vi "delme3.vi"() -> ()   [LabVIEW 2020]
uses:
  Project/GitInterface/Git-Repo JSON Typedef.ctl
panel:
  in  "Organization":string="P887"
  in  "Server":string="github.inbcu.com"
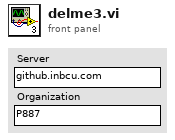
[diagram p1: front panel]
types:
  T1 = typedef "Git-Repo JSON Typedef.ctl" = cluster{"ID":string, "node_id":string, "name":string, "full_name":string, "private":string, "owner":string, "html_url":string, "description":string, "url":string, "collaborators_url":string, "teams_url":string}
  T2 = typedef "LabVIEWHTTPClient.lvlib/ClientHandle.ctl" = refnum<k1>
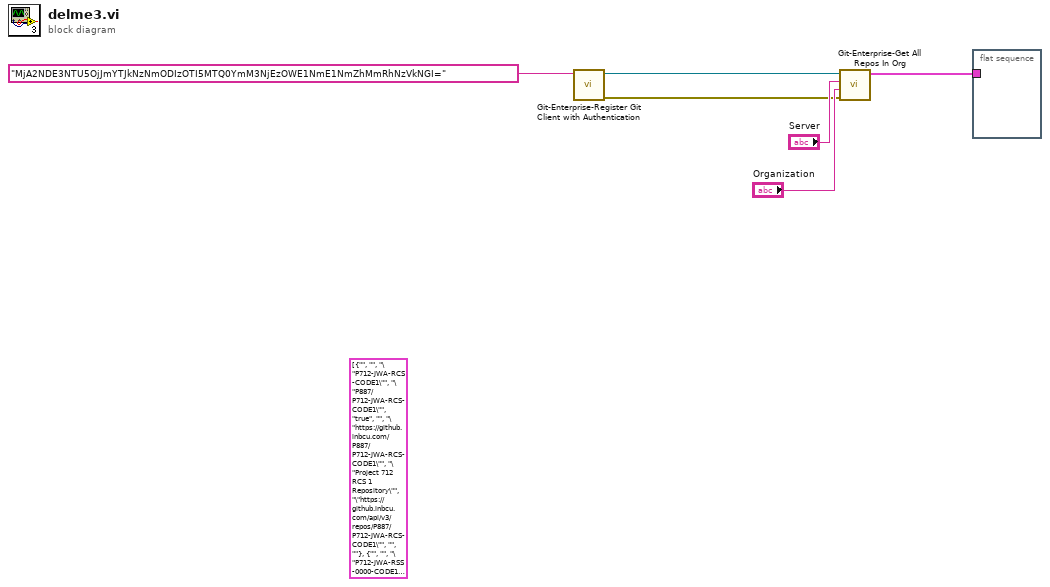
[diagram p0: block diagram]
diagram:
  (unwired) T1[] [{"ID"="", "node_id"="", "name"="\"P712-JWA-RCS-CODE1\"", "full_name"="\"P887/P712-JWA-RCS-CODE1\"", "private"="true", "owner"="", "html_url"="\"https://github.inbcu.com/P887/P712-JWA-RCS-CODE1\"", "description"="\"Project 712 RCS 1 Repository\"", "url"="\"https://github.inbcu.com/api/v3/repos/P887/P712-JWA-RCS-CODE1\"", "collaborators_url"="", "teams_url"=""}, {"ID"="", "node_id"="", "name"="\"P712-JWA-RSS-0000-CODE1\"", "full_name"="\"P887/P712-JWA-RSS-0000-CODE1\"", "private"="true", "owner"="", "html_url"="\"https://github.inbcu.com/P887/P712-JWA-RSS-0000-CODE1\"", "description"="\"RSS Software\"", "url"="\"https://github.inbcu.com/api/v3/repos/P887/P712-JWA-RSS-0000-CODE1\"", "collaborators_url"="", "teams_url"=""}, {"ID"="", "node_id"="", "name"="\"P714-KFP-RCS-CODE1\"", "full_name"="\"P887/P714-KFP-RCS-CODE1\"", "private"="true", "owner"="", "html_url"="\"https://github.inbcu.com/P887/P714-KFP-RCS-CODE1\"", "description"="\"KFP RCS Repository\"", "url"="\"https://github.inbcu.com/api/v3/repos/P887/P714-KFP-RCS-CODE1\"", "collaborators_url"="", "teams_url"=""}, {"ID"="", "node_id"="", "name"="\"P714-KFP-RSS-CODE1\"", "full_name"="\"P887/P714-KFP-RSS-CODE1\"", "private"="true", "owner"="", "html_url"="\"https://github.inbcu.com/P887/P714-KFP-RSS-CODE1\"", "description"="\"KFP RSS Software\"", "url"="\"https://github.inbcu.com/api/v3/repos/P887/P714-KFP-RSS-CODE1\"", "collaborators_url"="", "teams_url"=""}, {"ID"="", "node_id"="", "name"="\"P715-FJ-RCS-100-CODE1\"", "full_name"="\"P887/P715-FJ-RCS-100-CODE1\"", "private"="true", "owner"="", "html_url"="\"https://github.inbcu.com/P887/P715-FJ-RCS-100-CODE1\"", "description"="\"FJ RCS Software\"", "url"="\"https://github.inbcu.com/api/v3/repos/P887/P715-FJ-RCS-100-CODE1\"", "collaborators_url"="", "teams_url"=""}, {"ID"="", "node_id"="", "name"="\"P715-FJ-RSS-CODE1\"", "full_name"="\"P887/P715-FJ-RSS-CODE1\"", "private"="true", "owner"="", "html_url"="\"https://github.inbcu.com/P887/P715-FJ-RSS-CODE1\"", "description"="\"FJ RSS Software\"", "url"="\"https://github.inbcu.com/api/v3/repos/P887/P715-FJ-RSS-CODE1\"", "collaborators_url"="", "teams_url"=""}, {"ID"="", "node_id"="", "name"="\"P714-RIDE-AF-CODE1\"", "full_name"="\"P887/P714-RIDE-AF-CODE1\"", "private"="true", "owner"="", "html_url"="\"https://github.inbcu.com/P887/P714-RIDE-AF-CODE1\"", "description"="\"KFP Boat Ride SSC\"", "url"="\"https://github.inbcu.com/api/v3/repos/P887/P714-RIDE-AF-CODE1\"", "collaborators_url"="", "teams_url"=""}, {"ID"="", "node_id"="", "name"="\"P714-LAND-RSS-CODE1\"", "full_name"="\"P887/P714-LAND-RSS-CODE1\"", "private"="true", "owner"="", "html_url"="\"https://github.inbcu.com/P887/P714-LAND-RSS-CODE1\"", "description"="\"KFP Land RSS\"", "url"="\"https://github.inbcu.com/api/v3/repos/P887/P714-LAND-RSS-CODE1\"", "collaborators_url"="", "teams_url"=""}, {"ID"="", "node_id"="", "name"="\"P719-BARGE-SSC-CODE1\"", "full_name"="\"P887/P719-BARGE-SSC-CODE1\"", "private"="true", "owner"="", "html_url"="\"https://github.inbcu.com/P887/P719-BARGE-SSC-CODE1\"", "description"="\"Barge Controllers SSC\"", "url"="\"https://github.inbcu.com/api/v3/repos/P887/P719-BARGE-SSC-CODE1\"", "collaborators_url"="", "teams_url"=""}, {"ID"="", "node_id"="", "name"="\"LCA-RSS-CODE1\"", "full_name"="\"P887/LCA-RSS-CODE1\"", "private"="true", "owner"="", "html_url"="\"https://github.inbcu.com/P887/LCA-RSS-CODE1\"", "description"="\"LCA-RSS\"", "url"="\"https://github.inbcu.com/api/v3/repos/P887/LCA-RSS-CODE1\"", "collaborators_url"="", "teams_url"=""}, {"ID"="", "node_id"="", "name"="\"P717-COASTER-CODE1\"", "full_name"="\"P887/P717-COASTER-CODE1\"", "private"="true", "owner"="", "html_url"="\"https://github.inbcu.com/P887/P717-COASTER-CODE1\"", "description"="\"Pier Coaster RCS\"", "url"="\"https://github.inbcu.com/api/v3/repos/P887/P717-COASTER-CODE1\"", "collaborators_url"="", "teams_url"=""}, {"ID"="", "node_id"="", "name"="\"P717-PIER-ROUNDRIDE-CODE1\"", "full_name"="\"P887/P717-PIER-ROUNDRIDE-CODE1\"", "private"="true", "owner"="", "html_url"="\"https://github.inbcu.com/P887/P717-PIER-ROUNDRIDE-CODE1\"", "description"="\"P717 Pier Roundride\"", "url"="\"https://github.inbcu.com/api/v3/repos/P887/P717-PIER-ROUNDRIDE-CODE1\"", "collaborators_url"="", "teams_url"=""}, {"ID"="", "node_id"="", "name"="\"P717-MM-RCS-CODE1\"", "full_name"="\"P887/P717-MM-RCS-CODE1\"", "private"="true", "owner"="", "html_url"="\"https://github.inbcu.com/P887/P717-MM-RCS-CODE1\"", "description"="\"Minion Mayhem RCS Software\"", "url"="\"https://github.inbcu.com/api/v3/repos/P887/P717-MM-RCS-CODE1\"", "collaborators_url"="", "teams_url"=""}, {"ID"="", "node_id"="", "name"="\"P717-RSS-CODE1\"", "full_name"="\"P887/P717-RSS-CODE1\"", "private"="true", "owner"="", "html_url"="\"https://github.inbcu.com/P887/P717-RSS-CODE1\"", "description"="\"Minion Mayhem RSS Software\"", "url"="\"https://github.inbcu.com/api/v3/repos/P887/P717-RSS-CODE1\"", "collaborators_url"="", "teams_url"=""}, {"ID"="", "node_id"="", "name"="\"P717-HPU-CODE1\"", "full_name"="\"P887/P717-HPU-CODE1\"", "private"="true", "owner"="", "html_url"="\"https://github.inbcu.com/P887/P717-HPU-CODE1\"", "description"="\"Minion Mayhem HPU Software\"", "url"="\"https://github.inbcu.com/api/v3/repos/P887/P717-HPU-CODE1\"", "collaborators_url"="", "teams_url"=""}, {"ID"="", "node_id"="", "name"="\"P712-JFLYER-RCS-CODE1\"", "full_name"="\"P887/P712-JFLYER-RCS-CODE1\"", "private"="true", "owner"="", "html_url"="\"https://github.inbcu.com/P887/P712-JFLYER-RCS-CODE1\"", "description"="\"MACK Inverted Power Coaster\"", "url"="\"https://github.inbcu.com/api/v3/repos/P887/P712-JFLYER-RCS-CODE1\"", "collaborators_url"="", "teams_url"=""}, {"ID"="", "node_id"="", "name"="\"P716-TRANSFORMERS-RCS100-CODE1\"", "full_name"="\"P887/P716-TRANSFORMERS-RCS100-CODE1\"", "private"="true", "owner"="", "html_url"="\"https://github.inbcu.com/P887/P716-TRANSFORMERS-RCS100-CODE1\"", "description"="null", "url"="\"https://github.inbcu.com/api/v3/repos/P887/P716-TRANSFORMERS-RCS100-CODE1\"", "collaborators_url"="", "teams_url"=""}, {"ID"="", "node_id"="", "name"="\"P716-TRANSFORMERS-SSC400-CODE1\"", "full_name"="\"P887/P716-TRANSFORMERS-SSC400-CODE1\"", "private"="true", "owner"="", "html_url"="\"https://github.inbcu.com/P887/P716-TRANSFORMERS-SSC400-CODE1\"", "description"="null", "url"="\"https://github.inbcu.com/api/v3/repos/P887/P716-TRANSFORMERS-SSC400-CODE1\"", "collaborators_url"="", "teams_url"=""}, {"ID"="", "node_id"="", "name"="\"P716-TRANSFORMERS-SSC500-CODE1\"", "full_name"="\"P887/P716-TRANSFORMERS-SSC500-CODE1\"", "private"="true", "owner"="", "html_url"="\"https://github.inbcu.com/P887/P716-TRANSFORMERS-SSC500-CODE1\"", "description"="null", "url"="\"https://github.inbcu.com/api/v3/repos/P887/P716-TRANSFORMERS-SSC500-CODE1\"", "collaborators_url"="", "teams_url"=""}, {"ID"="", "node_id"="", "name"="\"P716-TRANSFORMERS-SSC600-CODE1\"", "full_name"="\"P887/P716-TRANSFORMERS-SSC600-CODE1\"", "private"="true", "owner"="", "html_url"="\"https://github.inbcu.com/P887/P716-TRANSFORMERS-SSC600-CODE1\"", "description"="null", "url"="\"https://github.inbcu.com/api/v3/repos/P887/P716-TRANSFORMERS-SSC600-CODE1\"", "collaborators_url"="", "teams_url"=""}, {"ID"="", "node_id"="", "name"="\"P716-TRANSFORMERS-SSC700-CODE1\"", "full_name"="\"P887/P716-TRANSFORMERS-SSC700-CODE1\"", "private"="true", "owner"="", "html_url"="\"https://github.inbcu.com/P887/P716-TRANSFORMERS-SSC700-CODE1\"", "description"="null", "url"="\"https://github.inbcu.com/api/v3/repos/P887/P716-TRANSFORMERS-SSC700-CODE1\"", "collaborators_url"="", "teams_url"=""}, {"ID"="", "node_id"="", "name"="\"P716-TRANSFORMERS-SSC800-CODE1\"", "full_name"="\"P887/P716-TRANSFORMERS-SSC800-CODE1\"", "private"="true", "owner"="", "html_url"="\"https://github.inbcu.com/P887/P716-TRANSFORMERS-SSC800-CODE1\"", "description"="null", "url"="\"https://github.inbcu.com/api/v3/repos/P887/P716-TRANSFORMERS-SSC800-CODE1\"", "collaborators_url"="", "teams_url"=""}, {"ID"="", "node_id"="", "name"="\"P716-TRANSFORMERS-SSC900-CODE1\"", "full_name"="\"P887/P716-TRANSFORMERS-SSC900-CODE1\"", "private"="true", "owner"="", "html_url"="\"https://github.inbcu.com/P887/P716-TRANSFORMERS-SSC900-CODE1\"", "description"="null", "url"="\"https://github.inbcu.com/api/v3/repos/P887/P716-TRANSFORMERS-SSC900-CODE1\"", "collaborators_url"="", "teams_url"=""}, {"ID"="", "node_id"="", "name"="\"P716-TRANSFORMERS-SSC1000-CODE1\"", "full_name"="\"P887/P716-TRANSFORMERS-SSC1000-CODE1\"", "private"="true", "owner"="", "html_url"="\"https://github.inbcu.com/P887/P716-TRANSFORMERS-SSC1000-CODE1\"", "description"="null", "url"="\"https://github.inbcu.com/api/v3/repos/P887/P716-TRANSFORMERS-SSC1000-CODE1\"", "collaborators_url"="", "teams_url"=""}, {"ID"="", "node_id"="", "name"="\"P716-TRANSFORMERS-SSC200-CODE1\"", "full_name"="\"P887/P716-TRANSFORMERS-SSC200-CODE1\"", "private"="true", "owner"="", "html_url"="\"https://github.inbcu.com/P887/P716-TRANSFORMERS-SSC200-CODE1\"", "description"="null", "url"="\"https://github.inbcu.com/api/v3/repos/P887/P716-TRANSFORMERS-SSC200-CODE1\"", "collaborators_url"="", "teams_url"=""}, {"ID"="", "node_id"="", "name"="\"P716-TRANSFORMERS-SSC300-CODE1\"", "full_name"="\"P887/P716-TRANSFORMERS-SSC300-CODE1\"", "private"="true", "owner"="", "html_url"="\"https://github.inbcu.com/P887/P716-TRANSFORMERS-SSC300-CODE1\"", "description"="null", "url"="\"https://github.inbcu.com/api/v3/repos/P887/P716-TRANSFORMERS-SSC300-CODE1\"", "collaborators_url"="", "teams_url"=""}, {"ID"="", "node_id"="", "name"="\"P715-LAND-LSS-CODE1\"", "full_name"="\"P887/P715-LAND-LSS-CODE1\"", "private"="true", "owner"="", "html_url"="\"https://github.inbcu.com/P887/P715-LAND-LSS-CODE1\"", "description"="null", "url"="\"https://github.inbcu.com/api/v3/repos/P887/P715-LAND-LSS-CODE1\"", "collaborators_url"="", "teams_url"=""}, {"ID"="", "node_id"="", "name"="\"P715-HIPPO-CODE1\"", "full_name"="\"P887/P715-HIPPO-CODE1\"", "private"="true", "owner"="", "html_url"="\"https://github.inbcu.com/P887/P715-HIPPO-CODE1\"", "description"="null", "url"="\"https://github.inbcu.com/api/v3/repos/P887/P715-HIPPO-CODE1\"", "collaborators_url"="", "teams_url"=""}, {"ID"="", "node_id"="", "name"="\"P711-FF-RCS-CODE1\"", "full_name"="\"P887/P711-FF-RCS-CODE1\"", "private"="true", "owner"="", "html_url"="\"https://github.inbcu.com/P887/P711-FF-RCS-CODE1\"", "description"="null", "url"="\"https://github.inbcu.com/api/v3/repos/P887/P711-FF-RCS-CODE1\"", "collaborators_url"="", "teams_url"=""}, {"ID"="", "node_id"="", "name"="\"P711-FF-RSS-CODE1\"", "full_name"="\"P887/P711-FF-RSS-CODE1\"", "private"="true", "owner"="", "html_url"="\"https://github.inbcu.com/P887/P711-FF-RSS-CODE1\"", "description"="null", "url"="\"https://github.inbcu.com/api/v3/repos/P887/P711-FF-RSS-CODE1\"", "collaborators_url"="", "teams_url"=""}, {"ID"="", "node_id"="", "name"="\"P712-JWA-RCS-CODE1\"", "full_name"="\"P887/P712-JWA-RCS-CODE1\"", "private"="true", "owner"="", "html_url"="\"https://github.inbcu.com/P887/P712-JWA-RCS-CODE1\"", "description"="\"Project 712 RCS 1 Repository\"", "url"="\"https://github.inbcu.com/api/v3/repos/P887/P712-JWA-RCS-CODE1\"", "collaborators_url"="", "teams_url"=""}, {"ID"="", "node_id"="", "name"="\"P712-JWA-RSS-0000-CODE1\"", "full_name"="\"P887/P712-JWA-RSS-0000-CODE1\"", "private"="true", "owner"="", "html_url"="\"https://github.inbcu.com/P887/P712-JWA-RSS-0000-CODE1\"", "description"="\"RSS Software\"", "url"="\"https://github.inbcu.com/api/v3/repos/P887/P712-JWA-RSS-0000-CODE1\"", "collaborators_url"="", "teams_url"=""}, {"ID"="", "node_id"="", "name"="\"P714-KFP-RCS-CODE1\"", "full_name"="\"P887/P714-KFP-RCS-CODE1\"", "private"="true", "owner"="", "html_url"="\"https://github.inbcu.com/P887/P714-KFP-RCS-CODE1\"", "description"="\"KFP RCS Repository\"", "url"="\"https://github.inbcu.com/api/v3/repos/P887/P714-KFP-RCS-CODE1\"", "collaborators_url"="", "teams_url"=""}, {"ID"="", "node_id"="", "name"="\"P714-KFP-RSS-CODE1\"", "full_name"="\"P887/P714-KFP-RSS-CODE1\"", "private"="true", "owner"="", "html_url"="\"https://github.inbcu.com/P887/P714-KFP-RSS-CODE1\"", "description"="\"KFP RSS Software\"", "url"="\"https://github.inbcu.com/api/v3/repos/P887/P714-KFP-RSS-CODE1\"", "collaborators_url"="", "teams_url"=""}, {"ID"="", "node_id"="", "name"="\"P715-FJ-RCS-100-CODE1\"", "full_name"="\"P887/P715-FJ-RCS-100-CODE1\"", "private"="true", "owner"="", "html_url"="\"https://github.inbcu.com/P887/P715-FJ-RCS-100-CODE1\"", "description"="\"FJ RCS Software\"", "url"="\"https://github.inbcu.com/api/v3/repos/P887/P715-FJ-RCS-100-CODE1\"", "collaborators_url"="", "teams_url"=""}, {"ID"="", "node_id"="", "name"="\"P715-FJ-RSS-CODE1\"", "full_name"="\"P887/P715-FJ-RSS-CODE1\"", "private"="true", "owner"="", "html_url"="\"https://github.inbcu.com/P887/P715-FJ-RSS-CODE1\"", "description"="\"FJ RSS Software\"", "url"="\"https://github.inbcu.com/api/v3/repos/P887/P715-FJ-RSS-CODE1\"", "collaborators_url"="", "teams_url"=""}, {"ID"="", "node_id"="", "name"="\"P714-RIDE-AF-CODE1\"", "full_name"="\"P887/P714-RIDE-AF-CODE1\"", "private"="true", "owner"="", "html_url"="\"https://github.inbcu.com/P887/P714-RIDE-AF-CODE1\"", "description"="\"KFP Boat Ride SSC\"", "url"="\"https://github.inbcu.com/api/v3/repos/P887/P714-RIDE-AF-CODE1\"", "collaborators_url"="", "teams_url"=""}, {"ID"="", "node_id"="", "name"="\"P714-LAND-RSS-CODE1\"", "full_name"="\"P887/P714-LAND-RSS-CODE1\"", "private"="true", "owner"="", "html_url"="\"https://github.inbcu.com/P887/P714-LAND-RSS-CODE1\"", "description"="\"KFP Land RSS\"", "url"="\"https://github.inbcu.com/api/v3/repos/P887/P714-LAND-RSS-CODE1\"", "collaborators_url"="", "teams_url"=""}, {"ID"="", "node_id"="", "name"="\"P719-BARGE-SSC-CODE1\"", "full_name"="\"P887/P719-BARGE-SSC-CODE1\"", "private"="true", "owner"="", "html_url"="\"https://github.inbcu.com/P887/P719-BARGE-SSC-CODE1\"", "description"="\"Barge Controllers SSC\"", "url"="\"https://github.inbcu.com/api/v3/repos/P887/P719-BARGE-SSC-CODE1\"", "collaborators_url"="", "teams_url"=""}, {"ID"="", "node_id"="", "name"="\"LCA-RSS-CODE1\"", "full_name"="\"P887/LCA-RSS-CODE1\"", "private"="true", "owner"="", "html_url"="\"https://github.inbcu.com/P887/LCA-RSS-CODE1\"", "description"="\"LCA-RSS\"", "url"="\"https://github.inbcu.com/api/v3/repos/P887/LCA-RSS-CODE1\"", "collaborators_url"="", "teams_url"=""}, {"ID"="", "node_id"="", "name"="\"P717-COASTER-CODE1\"", "full_name"="\"P887/P717-COASTER-CODE1\"", "private"="true", "owner"="", "html_url"="\"https://github.inbcu.com/P887/P717-COASTER-CODE1\"", "description"="\"Pier Coaster RCS\"", "url"="\"https://github.inbcu.com/api/v3/repos/P887/P717-COASTER-CODE1\"", "collaborators_url"="", "teams_url"=""}, {"ID"="", "node_id"="", "name"="\"P717-PIER-ROUNDRIDE-CODE1\"", "full_name"="\"P887/P717-PIER-ROUNDRIDE-CODE1\"", "private"="true", "owner"="", "html_url"="\"https://github.inbcu.com/P887/P717-PIER-ROUNDRIDE-CODE1\"", "description"="\"P717 Pier Roundride\"", "url"="\"https://github.inbcu.com/api/v3/repos/P887/P717-PIER-ROUNDRIDE-CODE1\"", "collaborators_url"="", "teams_url"=""}, {"ID"="", "node_id"="", "name"="\"P717-MM-RCS-CODE1\"", "full_name"="\"P887/P717-MM-RCS-CODE1\"", "private"="true", "owner"="", "html_url"="\"https://github.inbcu.com/P887/P717-MM-RCS-CODE1\"", "description"="\"Minion Mayhem RCS Software\"", "url"="\"https://github.inbcu.com/api/v3/repos/P887/P717-MM-RCS-CODE1\"", "collaborators_url"="", "teams_url"=""}, {"ID"="", "node_id"="", "name"="\"P717-RSS-CODE1\"", "full_name"="\"P887/P717-RSS-CODE1\"", "private"="true", "owner"="", "html_url"="\"https://github.inbcu.com/P887/P717-RSS-CODE1\"", "description"="\"Minion Mayhem RSS Software\"", "url"="\"https://github.inbcu.com/api/v3/repos/P887/P717-RSS-CODE1\"", "collaborators_url"="", "teams_url"=""}, {"ID"="", "node_id"="", "name"="\"P717-HPU-CODE1\"", "full_name"="\"P887/P717-HPU-CODE1\"", "private"="true", "owner"="", "html_url"="\"https://github.inbcu.com/P887/P717-HPU-CODE1\"", "description"="\"Minion Mayhem HPU Software\"", "url"="\"https://github.inbcu.com/api/v3/repos/P887/P717-HPU-CODE1\"", "collaborators_url"="", "teams_url"=""}, {"ID"="", "node_id"="", "name"="\"P712-JFLYER-RCS-CODE1\"", "full_name"="\"P887/P712-JFLYER-RCS-CODE1\"", "private"="true", "owner"="", "html_url"="\"https://github.inbcu.com/P887/P712-JFLYER-RCS-CODE1\"", "description"="\"MACK Inverted Power Coaster\"", "url"="\"https://github.inbcu.com/api/v3/repos/P887/P712-JFLYER-RCS-CODE1\"", "collaborators_url"="", "teams_url"=""}, {"ID"="", "node_id"="", "name"="\"P716-TRANSFORMERS-RCS100-CODE1\"", "full_name"="\"P887/P716-TRANSFORMERS-RCS100-CODE1\"", "private"="true", "owner"="", "html_url"="\"https://github.inbcu.com/P887/P716-TRANSFORMERS-RCS100-CODE1\"", "description"="null", "url"="\"https://github.inbcu.com/api/v3/repos/P887/P716-TRANSFORMERS-RCS100-CODE1\"", "collaborators_url"="", "teams_url"=""}, {"ID"="", "node_id"="", "name"="\"P716-TRANSFORMERS-SSC400-CODE1\"", "full_name"="\"P887/P716-TRANSFORMERS-SSC400-CODE1\"", "private"="true", "owner"="", "html_url"="\"https://github.inbcu.com/P887/P716-TRANSFORMERS-SSC400-CODE1\"", "description"="null", "url"="\"https://github.inbcu.com/api/v3/repos/P887/P716-TRANSFORMERS-SSC400-CODE1\"", "collaborators_url"="", "teams_url"=""}, {"ID"="", "node_id"="", "name"="\"P716-TRANSFORMERS-SSC500-CODE1\"", "full_name"="\"P887/P716-TRANSFORMERS-SSC500-CODE1\"", "private"="true", "owner"="", "html_url"="\"https://github.inbcu.com/P887/P716-TRANSFORMERS-SSC500-CODE1\"", "description"="null", "url"="\"https://github.inbcu.com/api/v3/repos/P887/P716-TRANSFORMERS-SSC500-CODE1\"", "collaborators_url"="", "teams_url"=""}, {"ID"="", "node_id"="", "name"="\"P716-TRANSFORMERS-SSC600-CODE1\"", "full_name"="\"P887/P716-TRANSFORMERS-SSC600-CODE1\"", "private"="true", "owner"="", "html_url"="\"https://github.inbcu.com/P887/P716-TRANSFORMERS-SSC600-CODE1\"", "description"="null", "url"="\"https://github.inbcu.com/api/v3/repos/P887/P716-TRANSFORMERS-SSC600-CODE1\"", "collaborators_url"="", "teams_url"=""}, {"ID"="", "node_id"="", "name"="\"P716-TRANSFORMERS-SSC700-CODE1\"", "full_name"="\"P887/P716-TRANSFORMERS-SSC700-CODE1\"", "private"="true", "owner"="", "html_url"="\"https://github.inbcu.com/P887/P716-TRANSFORMERS-SSC700-CODE1\"", "description"="null", "url"="\"https://github.inbcu.com/api/v3/repos/P887/P716-TRANSFORMERS-SSC700-CODE1\"", "collaborators_url"="", "teams_url"=""}, {"ID"="", "node_id"="", "name"="\"P716-TRANSFORMERS-SSC800-CODE1\"", "full_name"="\"P887/P716-TRANSFORMERS-SSC800-CODE1\"", "private"="true", "owner"="", "html_url"="\"https://github.inbcu.com/P887/P716-TRANSFORMERS-SSC800-CODE1\"", "description"="null", "url"="\"https://github.inbcu.com/api/v3/repos/P887/P716-TRANSFORMERS-SSC800-CODE1\"", "collaborators_url"="", "teams_url"=""}, {"ID"="", "node_id"="", "name"="\"P716-TRANSFORMERS-SSC900-CODE1\"", "full_name"="\"P887/P716-TRANSFORMERS-SSC900-CODE1\"", "private"="true", "owner"="", "html_url"="\"https://github.inbcu.com/P887/P716-TRANSFORMERS-SSC900-CODE1\"", "description"="null", "url"="\"https://github.inbcu.com/api/v3/repos/P887/P716-TRANSFORMERS-SSC900-CODE1\"", "collaborators_url"="", "teams_url"=""}, {"ID"="", "node_id"="", "name"="\"P716-TRANSFORMERS-SSC1000-CODE1\"", "full_name"="\"P887/P716-TRANSFORMERS-SSC1000-CODE1\"", "private"="true", "owner"="", "html_url"="\"https://github.inbcu.com/P887/P716-TRANSFORMERS-SSC1000-CODE1\"", "description"="null", "url"="\"https://github.inbcu.com/api/v3/repos/P887/P716-TRANSFORMERS-SSC1000-CODE1\"", "collaborators_url"="", "teams_url"=""}, {"ID"="", "node_id"="", "name"="\"P716-TRANSFORMERS-SSC200-CODE1\"", "full_name"="\"P887/P716-TRANSFORMERS-SSC200-CODE1\"", "private"="true", "owner"="", "html_url"="\"https://github.inbcu.com/P887/P716-TRANSFORMERS-SSC200-CODE1\"", "description"="null", "url"="\"https://github.inbcu.com/api/v3/repos/P887/P716-TRANSFORMERS-SSC200-CODE1\"", "collaborators_url"="", "teams_url"=""}, {"ID"="", "node_id"="", "name"="\"P716-TRANSFORMERS-SSC300-CODE1\"", "full_name"="\"P887/P716-TRANSFORMERS-SSC300-CODE1\"", "private"="true", "owner"="", "html_url"="\"https://github.inbcu.com/P887/P716-TRANSFORMERS-SSC300-CODE1\"", "description"="null", "url"="\"https://github.inbcu.com/api/v3/repos/P887/P716-TRANSFORMERS-SSC300-CODE1\"", "collaborators_url"="", "teams_url"=""}, {"ID"="", "node_id"="", "name"="\"P715-LAND-LSS-CODE1\"", "full_name"="\"P887/P715-LAND-LSS-CODE1\"", "private"="true", "owner"="", "html_url"="\"https://github.inbcu.com/P887/P715-LAND-LSS-CODE1\"", "description"="null", "url"="\"https://github.inbcu.com/api/v3/repos/P887/P715-LAND-LSS-CODE1\"", "collaborators_url"="", "teams_url"=""}, {"ID"="", "node_id"="", "name"="\"P715-HIPPO-CODE1\"", "full_name"="\"P887/P715-HIPPO-CODE1\"", "private"="true", "owner"="", "html_url"="\"https://github.inbcu.com/P887/P715-HIPPO-CODE1\"", "description"="null", "url"="\"https://github.inbcu.com/api/v3/repos/P887/P715-HIPPO-CODE1\"", "collaborators_url"="", "teams_url"=""}, {"ID"="", "node_id"="", "name"="\"P711-FF-RCS-CODE1\"", "full_name"="\"P887/P711-FF-RCS-CODE1\"", "private"="true", "owner"="", "html_url"="\"https://github.inbcu.com/P887/P711-FF-RCS-CODE1\"", "description"="null", "url"="\"https://github.inbcu.com/api/v3/repos/P887/P711-FF-RCS-CODE1\"", "collaborators_url"="", "teams_url"=""}, {"ID"="", "node_id"="", "name"="\"P711-FF-RSS-CODE1\"", "full_name"="\"P887/P711-FF-RSS-CODE1\"", "private"="true", "owner"="", "html_url"="\"https://github.inbcu.com/P887/P711-FF-RSS-CODE1\"", "description"="null", "url"="\"https://github.inbcu.com/api/v3/repos/P887/P711-FF-RSS-CODE1\"", "collaborators_url"="", "teams_url"=""}, {"ID"="", "node_id"="", "name"="\"P711-FF-HPU-CODE1\"", "full_name"="\"P887/P711-FF-HPU-CODE1\"", "private"="true", "owner"="", "html_url"="\"https://github.inbcu.com/P887/P711-FF-HPU-CODE1\"", "description"="null", "url"="\"https://github.inbcu.com/api/v3/repos/P887/P711-FF-HPU-CODE1\"", "collaborators_url"="", "teams_url"=""}, {"ID"="", "node_id"="", "name"="\"P711-FF-RVMV-CODE1\"", "full_name"="\"P887/P711-FF-RVMV-CODE1\"", "private"="true", "owner"="", "html_url"="\"https://github.inbcu.com/P887/P711-FF-RVMV-CODE1\"", "description"="null", "url"="\"https://github.inbcu.com/api/v3/repos/P887/P711-FF-RVMV-CODE1\"", "collaborators_url"="", "teams_url"=""}, {"ID"="", "node_id"="", "name"="\"P711-FF-SD-CODE1\"", "full_name"="\"P887/P711-FF-SD-CODE1\"", "private"="true", "owner"="", "html_url"="\"https://github.inbcu.com/P887/P711-FF-SD-CODE1\"", "description"="null", "url"="\"https://github.inbcu.com/api/v3/repos/P887/P711-FF-SD-CODE1\"", "collaborators_url"="", "teams_url"=""}, {"ID"="", "node_id"="", "name"="\"P711-FF-FS-CODE1\"", "full_name"="\"P887/P711-FF-FS-CODE1\"", "private"="true", "owner"="", "html_url"="\"https://github.inbcu.com/P887/P711-FF-FS-CODE1\"", "description"="\"Flying Screen\"", "url"="\"https://github.inbcu.com/api/v3/repos/P887/P711-FF-FS-CODE1\"", "collaborators_url"="", "teams_url"=""}, {"ID"="", "node_id"="", "name"="\"P711-FF-LN2-CODE1\"", "full_name"="\"P887/P711-FF-LN2-CODE1\"", "private"="true", "owner"="", "html_url"="\"https://github.inbcu.com/P887/P711-FF-LN2-CODE1\"", "description"="\"LN2\"", "url"="\"https://github.inbcu.com/api/v3/repos/P887/P711-FF-LN2-CODE1\"", "collaborators_url"="", "teams_url"=""}, {"ID"="", "node_id"="", "name"="\"P711-LCA-RSS100-CODE1\"", "full_name"="\"P887/P711-LCA-RSS100-CODE1\"", "private"="true", "owner"="", "html_url"="\"https://github.inbcu.com/P887/P711-LCA-RSS100-CODE1\"", "description"="null", "url"="\"https://github.inbcu.com/api/v3/repos/P887/P711-LCA-RSS100-CODE1\"", "collaborators_url"="", "teams_url"=""}, {"ID"="", "node_id"="", "name"="\"P711-MPT-RSS-CODE1\"", "full_name"="\"P887/P711-MPT-RSS-CODE1\"", "private"="true", "owner"="", "html_url"="\"https://github.inbcu.com/P887/P711-MPT-RSS-CODE1\"", "description"="null", "url"="\"https://github.inbcu.com/api/v3/repos/P887/P711-MPT-RSS-CODE1\"", "collaborators_url"="", "teams_url"=""}, {"ID"="", "node_id"="", "name"="\"P719-LAGOON-RSS-CODE1\"", "full_name"="\"P887/P719-LAGOON-RSS-CODE1\"", "private"="true", "owner"="", "html_url"="\"https://github.inbcu.com/P887/P719-LAGOON-RSS-CODE1\"", "description"="\"Lagoon Show RSS\"", "url"="\"https://github.inbcu.com/api/v3/repos/P887/P719-LAGOON-RSS-CODE1\"", "collaborators_url"="", "teams_url"=""}, {"ID"="", "node_id"="", "name"="\"P716-ROUNDRIDE-CODE1\"", "full_name"="\"P887/P716-ROUNDRIDE-CODE1\"", "private"="true", "owner"="", "html_url"="\"https://github.inbcu.com/P887/P716-ROUNDRIDE-CODE1\"", "description"="\"Transformers base Bumblebee Boogie Round Ride\"", "url"="\"https://github.inbcu.com/api/v3/repos/P887/P716-ROUNDRIDE-CODE1\"", "collaborators_url"="", "teams_url"=""}, {"ID"="", "node_id"="", "name"="\"P716-BBAF-CODE1\"", "full_name"="\"P887/P716-BBAF-CODE1\"", "private"="true", "owner"="", "html_url"="\"https://github.inbcu.com/P887/P716-BBAF-CODE1\"", "description"="\"Transformers Base Bumblebee Boogie Animated Figure\"", "url"="\"https://github.inbcu.com/api/v3/repos/P887/P716-BBAF-CODE1\"", "collaborators_url"="", "teams_url"=""}, {"ID"="", "node_id"="", "name"="\"P716-DECEPTICOASTER-RCS-CODE1\"", "full_name"="\"P887/P716-DECEPTICOASTER-RCS-CODE1\"", "private"="true", "owner"="", "html_url"="\"https://github.inbcu.com/P887/P716-DECEPTICOASTER-RCS-CODE1\"", "description"="\"Decepticoaster Ride System \"", "url"="\"https://github.inbcu.com/api/v3/repos/P887/P716-DECEPTICOASTER-RCS-CODE1\"", "collaborators_url"="", "teams_url"=""}, {"ID"="", "node_id"="", "name"="\"P714-12ARM-CODE1\"", "full_name"="\"P887/P714-12ARM-CODE1\"", "private"="true", "owner"="", "html_url"="\"https://github.inbcu.com/P887/P714-12ARM-CODE1\"", "description"="\"KFP Land 12 arm round ride\"", "url"="\"https://github.inbcu.com/api/v3/repos/P887/P714-12ARM-CODE1\"", "collaborators_url"="", "teams_url"=""}, {"ID"="", "node_id"="", "name"="\"P714-CAROUSEL-CODE1\"", "full_name"="\"P887/P714-CAROUSEL-CODE1\"", "private"="true", "owner"="", "html_url"="\"https://github.inbcu.com/P887/P714-CAROUSEL-CODE1\"", "description"="\"KFP Land Carousel Ride System\"", "url"="\"https://github.inbcu.com/api/v3/repos/P887/P714-CAROUSEL-CODE1\"", "collaborators_url"="", "teams_url"=""}, {"ID"="", "node_id"="", "name"="\"P716-DECEPTICOASTER-RSS-CODE1\"", "full_name"="\"P887/P716-DECEPTICOASTER-RSS-CODE1\"", "private"="true", "owner"="", "html_url"="\"https://github.inbcu.com/P887/P716-DECEPTICOASTER-RSS-CODE1\"", "description"="\"Transformers Decepticoaster RSS System\"", "url"="\"https://github.inbcu.com/api/v3/repos/P887/P716-DECEPTICOASTER-RSS-CODE1\"", "collaborators_url"="", "teams_url"=""}, {"ID"="", "node_id"="", "name"="\"P716-TRANSFORMERS-RSS-CODE1\"", "full_name"="\"P887/P716-TRANSFORMERS-RSS-CODE1\"", "private"="true", "owner"="", "html_url"="\"https://github.inbcu.com/P887/P716-TRANSFORMERS-RSS-CODE1\"", "description"="\"Transformers Ride RSS System\"", "url"="\"https://github.inbcu.com/api/v3/repos/P887/P716-TRANSFORMERS-RSS-CODE1\"", "collaborators_url"="", "teams_url"=""}, {"ID"="", "node_id"="", "name"="\"P715-FJ-RCS-200-CODE1\"", "full_name"="\"P887/P715-FJ-RCS-200-CODE1\"", "private"="true", "owner"="", "html_url"="\"https://github.inbcu.com/P887/P715-FJ-RCS-200-CODE1\"", "description"="null", "url"="\"https://github.inbcu.com/api/v3/repos/P887/P715-FJ-RCS-200-CODE1\"", "collaborators_url"="", "teams_url"=""}, {"ID"="", "node_id"="", "name"="\"P715-FJ-RCS-300-CODE1\"", "full_name"="\"P887/P715-FJ-RCS-300-CODE1\"", "private"="true", "owner"="", "html_url"="\"https://github.inbcu.com/P887/P715-FJ-RCS-300-CODE1\"", "description"="null", "url"="\"https://github.inbcu.com/api/v3/repos/P887/P715-FJ-RCS-300-CODE1\"", "collaborators_url"="", "teams_url"=""}, {"ID"="", "node_id"="", "name"="\"P715-FJ-RCS-400-CODE1\"", "full_name"="\"P887/P715-FJ-RCS-400-CODE1\"", "private"="true", "owner"="", "html_url"="\"https://github.inbcu.com/P887/P715-FJ-RCS-400-CODE1\"", "description"="\"TT (TT1 and TT2)\"", "url"="\"https://github.inbcu.com/api/v3/repos/P887/P715-FJ-RCS-400-CODE1\"", "collaborators_url"="", "teams_url"=""}, {"ID"="", "node_id"="", "name"="\"P715-FJ-RCS-500-CODE1\"", "full_name"="\"P887/P715-FJ-RCS-500-CODE1\"", "private"="true", "owner"="", "html_url"="\"https://github.inbcu.com/P887/P715-FJ-RCS-500-CODE1\"", "description"="\"PM (magic carpet)\"", "url"="\"https://github.inbcu.com/api/v3/repos/P887/P715-FJ-RCS-500-CODE1\"", "collaborators_url"="", "teams_url"=""}, {"ID"="", "node_id"="", "name"="\"P715-FJ-RCS-600-CODE1\"", "full_name"="\"P887/P715-FJ-RCS-600-CODE1\"", "private"="true", "owner"="", "html_url"="\"https://github.inbcu.com/P887/P715-FJ-RCS-600-CODE1\"", "description"="\"WSS\"", "url"="\"https://github.inbcu.com/api/v3/repos/P887/P715-FJ-RCS-600-CODE1\"", "collaborators_url"="", "teams_url"=""}, {"ID"="", "node_id"="", "name"="\"P715-FJ-VCS-1-CODE1\"", "full_name"="\"P887/P715-FJ-VCS-1-CODE1\"", "private"="true", "owner"="", "html_url"="\"https://github.inbcu.com/P887/P715-FJ-VCS-1-CODE1\"", "description"="\"VCS 1\"", "url"="\"https://github.inbcu.com/api/v3/repos/P887/P715-FJ-VCS-1-CODE1\"", "collaborators_url"="", "teams_url"=""}, {"ID"="", "node_id"="", "name"="\"P715-FJ-SSC-700-CODE1\"", "full_name"="\"P887/P715-FJ-SSC-700-CODE1\"", "private"="true", "owner"="", "html_url"="\"https://github.inbcu.com/P887/P715-FJ-SSC-700-CODE1\"", "description"="\"Carousel 1\"", "url"="\"https://github.inbcu.com/api/v3/repos/P887/P715-FJ-SSC-700-CODE1\"", "collaborators_url"="", "teams_url"=""}, {"ID"="", "node_id"="", "name"="\"P715-FJ-SSC-800-CODE1\"", "full_name"="\"P887/P715-FJ-SSC-800-CODE1\"", "private"="true", "owner"="", "html_url"="\"https://github.inbcu.com/P887/P715-FJ-SSC-800-CODE1\"", "description"="\"Carousel 2\"", "url"="\"https://github.inbcu.com/api/v3/repos/P887/P715-FJ-SSC-800-CODE1\"", "collaborators_url"="", "teams_url"=""}, {"ID"="", "node_id"="", "name"="\"P715-FJ-SSC-900-CODE1\"", "full_name"="\"P887/P715-FJ-SSC-900-CODE1\"", "private"="true", "owner"="", "html_url"="\"https://github.inbcu.com/P887/P715-FJ-SSC-900-CODE1\"", "description"="\"Carousel 3\"", "url"="\"https://github.inbcu.com/api/v3/repos/P887/P715-FJ-SSC-900-CODE1\"", "collaborators_url"="", "teams_url"=""}, {"ID"="", "node_id"="", "name"="\"P715-FJ-SSC-1000-CODE1\"", "full_name"="\"P887/P715-FJ-SSC-1000-CODE1\"", "private"="true", "owner"="", "html_url"="\"https://github.inbcu.com/P887/P715-FJ-SSC-1000-CODE1\"", "description"="\"Dementor Willow SAE\"", "url"="\"https://github.inbcu.com/api/v3/repos/P887/P715-FJ-SSC-1000-CODE1\"", "collaborators_url"="", "teams_url"=""}, {"ID"="", "node_id"="", "name"="\"P715-FJ-SSC-2100-CODE1\"", "full_name"="\"P887/P715-FJ-SSC-2100-CODE1\"", "private"="true", "owner"="", "html_url"="\"https://github.inbcu.com/P887/P715-FJ-SSC-2100-CODE1\"", "description"="\"Dragon\"", "url"="\"https://github.inbcu.com/api/v3/repos/P887/P715-FJ-SSC-2100-CODE1\"", "collaborators_url"="", "teams_url"=""}, {"ID"="", "node_id"="", "name"="\"P715-FJ-SSC-1200-CODE1\"", "full_name"="\"P887/P715-FJ-SSC-1200-CODE1\"", "private"="true", "owner"="", "html_url"="\"https://github.inbcu.com/P887/P715-FJ-SSC-1200-CODE1\"", "description"="\"Scene 1 - 7 Special Effects\"", "url"="\"https://github.inbcu.com/api/v3/repos/P887/P715-FJ-SSC-1200-CODE1\"", "collaborators_url"="", "teams_url"=""}, {"ID"="", "node_id"="", "name"="\"P715-FJ-SSC-1300-CODE1\"", "full_name"="\"P887/P715-FJ-SSC-1300-CODE1\"", "private"="true", "owner"="", "html_url"="\"https://github.inbcu.com/P887/P715-FJ-SSC-1300-CODE1\"", "description"="\"Scene 8-11 Special Effects\"", "url"="\"https://github.inbcu.com/api/v3/repos/P887/P715-FJ-SSC-1300-CODE1\"", "collaborators_url"="", "teams_url"=""}, {"ID"="", "node_id"="", "name"="\"P712-JWA-TS-CODE1\"", "full_name"="\"P887/P712-JWA-TS-CODE1\"", "private"="true", "owner"="", "html_url"="\"https://github.inbcu.com/P887/P712-JWA-TS-CODE1\"", "description"="\"JW TS RCS 200\"", "url"="\"https://github.inbcu.com/api/v3/repos/P887/P712-JWA-TS-CODE1\"", "collaborators_url"="", "teams_url"=""}, {"ID"="", "node_id"="", "name"="\"P712-JWA-SSC-2100-IREX1-CODE1\"", "full_name"="\"P887/P712-JWA-SSC-2100-IREX1-CODE1\"", "private"="true", "owner"="", "html_url"="\"https://github.inbcu.com/P887/P712-JWA-SSC-2100-IREX1-CODE1\"", "description"="\"JW Large AF SSC 2100\"", "url"="\"https://github.inbcu.com/api/v3/repos/P887/P712-JWA-SSC-2100-IREX1-CODE1\"", "collaborators_url"="", "teams_url"=""}, {"ID"="", "node_id"="", "name"="\"P712-JWA-SSC-2200-Anky-CODE1\"", "full_name"="\"P887/P712-JWA-SSC-2200-Anky-CODE1\"", "private"="true", "owner"="", "html_url"="\"https://github.inbcu.com/P887/P712-JWA-SSC-2200-Anky-CODE1\"", "description"="\"JW Large AF SSC 2200\"", "url"="\"https://github.inbcu.com/api/v3/repos/P887/P712-JWA-SSC-2200-Anky-CODE1\"", "collaborators_url"="", "teams_url"=""}, {"ID"="", "node_id"="", "name"="\"P712-JWA-SSC-2300-IREX2-CODE1\"", "full_name"="\"P887/P712-JWA-SSC-2300-IREX2-CODE1\"", "private"="true", "owner"="", "html_url"="\"https://github.inbcu.com/P887/P712-JWA-SSC-2300-IREX2-CODE1\"", "description"="\"JW Large AF SSC 2300\"", "url"="\"https://github.inbcu.com/api/v3/repos/P887/P712-JWA-SSC-2300-IREX2-CODE1\"", "collaborators_url"="", "teams_url"=""}, {"ID"="", "node_id"="", "name"="\"P712-JWA-SSC-2700-IREX3-CODE1\"", "full_name"="\"P887/P712-JWA-SSC-2700-IREX3-CODE1\"", "private"="true", "owner"="", "html_url"="\"https://github.inbcu.com/P887/P712-JWA-SSC-2700-IREX3-CODE1\"", "description"="\"JW Large AF SSC 2700\"", "url"="\"https://github.inbcu.com/api/v3/repos/P887/P712-JWA-SSC-2700-IREX3-CODE1\"", "collaborators_url"="", "teams_url"=""}, {"ID"="", "node_id"="", "name"="\"P712-JWA-SSC-2800-TREX-CODE1\"", "full_name"="\"P887/P712-JWA-SSC-2800-TREX-CODE1\"", "private"="true", "owner"="", "html_url"="\"https://github.inbcu.com/P887/P712-JWA-SSC-2800-TREX-CODE1\"", "description"="\"JW Large AF SSC 2800\"", "url"="\"https://github.inbcu.com/api/v3/repos/P887/P712-JWA-SSC-2800-TREX-CODE1\"", "collaborators_url"="", "teams_url"=""}, {"ID"="", "node_id"="", "name"="\"P712-JWA-SSC-2900-FH-CODE1\"", "full_name"="\"P887/P712-JWA-SSC-2900-FH-CODE1\"", "private"="true", "owner"="", "html_url"="\"https://github.inbcu.com/P887/P712-JWA-SSC-2900-FH-CODE1\"", "description"="\"JW Large AF SSC 2900\"", "url"="\"https://github.inbcu.com/api/v3/repos/P887/P712-JWA-SSC-2900-FH-CODE1\"", "collaborators_url"="", "teams_url"=""}, {"ID"="", "node_id"="", "name"="\"P712-JW-SSC-2400-CODE1\"", "full_name"="\"P887/P712-JW-SSC-2400-CODE1\"", "private"="true", "owner"="", "html_url"="\"https://github.inbcu.com/P887/P712-JW-SSC-2400-CODE1\"", "description"="\"JW SAE\"", "url"="\"https://github.inbcu.com/api/v3/repos/P887/P712-JW-SSC-2400-CODE1\"", "collaborators_url"="", "teams_url"=""}, {"ID"="", "node_id"="", "name"="\"P712-JW-SSC-2600-CODE1\"", "full_name"="\"P887/P712-JW-SSC-2600-CODE1\"", "private"="true", "owner"="", "html_url"="\"https://github.inbcu.com/P887/P712-JW-SSC-2600-CODE1\"", "description"="\"JW Raptor\"", "url"="\"https://github.inbcu.com/api/v3/repos/P887/P712-JW-SSC-2600-CODE1\"", "collaborators_url"="", "teams_url"=""}, {"ID"="", "node_id"="", "name"="\"P712-JW-SSC-2500-CODE1\"", "full_name"="\"P887/P712-JW-SSC-2500-CODE1\"", "private"="true", "owner"="", "html_url"="\"https://github.inbcu.com/P887/P712-JW-SSC-2500-CODE1\"", "description"="\"JW SA\"", "url"="\"https://github.inbcu.com/api/v3/repos/P887/P712-JW-SSC-2500-CODE1\"", "collaborators_url"="", "teams_url"=""}, {"ID"="", "node_id"="", "name"="\"P712-JWA-SCS-2000-CODE1\"", "full_name"="\"P887/P712-JWA-SCS-2000-CODE1\"", "private"="true", "owner"="", "html_url"="\"https://github.inbcu.com/P887/P712-JWA-SCS-2000-CODE1\"", "description"="\"JW SCS\"", "url"="\"https://github.inbcu.com/api/v3/repos/P887/P712-JWA-SCS-2000-CODE1\"", "collaborators_url"="", "teams_url"=""}, {"ID"="", "node_id"="", "name"="\"P712-JWA-VCS-CODE1\"", "full_name"="\"P887/P712-JWA-VCS-CODE1\"", "private"="true", "owner"="", "html_url"="\"https://github.inbcu.com/P887/P712-JWA-VCS-CODE1\"", "description"="\"JW VCS 1\"", "url"="\"https://github.inbcu.com/api/v3/repos/P887/P712-JWA-VCS-CODE1\"", "collaborators_url"="", "teams_url"=""}, {"ID"="", "node_id"="", "name"="\"P711-LCA-SSC200-CODE1\"", "full_name"="\"P887/P711-LCA-SSC200-CODE1\"", "private"="true", "owner"="", "html_url"="\"https://github.inbcu.com/P887/P711-LCA-SSC200-CODE1\"", "description"="\"Lights Camera Action SAE/SFX SSC\"", "url"="\"https://github.inbcu.com/api/v3/repos/P887/P711-LCA-SSC200-CODE1\"", "collaborators_url"="", "teams_url"=""}, {"ID"="", "node_id"="", "name"="\"P711-LCA-SSC300-CODE1\"", "full_name"="\"P887/P711-LCA-SSC300-CODE1\"", "private"="true", "owner"="", "html_url"="\"https://github.inbcu.com/P887/P711-LCA-SSC300-CODE1\"", "description"="\"Lights Camera Action SAE/SFX SSC\"", "url"="\"https://github.inbcu.com/api/v3/repos/P887/P711-LCA-SSC300-CODE1\"", "collaborators_url"="", "teams_url"=""}, {"ID"="", "node_id"="", "name"="\"P711-LCA-SSC400-CODE1\"", "full_name"="\"P887/P711-LCA-SSC400-CODE1\"", "private"="true", "owner"="", "html_url"="\"https://github.inbcu.com/P887/P711-LCA-SSC400-CODE1\"", "description"="\"Lights Camera Action SAE/SFX SSC\"", "url"="\"https://github.inbcu.com/api/v3/repos/P887/P711-LCA-SSC400-CODE1\"", "collaborators_url"="", "teams_url"=""}, {"ID"="", "node_id"="", "name"="\"P711-LCA-SSC500-CODE1\"", "full_name"="\"P887/P711-LCA-SSC500-CODE1\"", "private"="true", "owner"="", "html_url"="\"https://github.inbcu.com/P887/P711-LCA-SSC500-CODE1\"", "description"="\"Lights Camera Action SAE/SFX SSC\"", "url"="\"https://github.inbcu.com/api/v3/repos/P887/P711-LCA-SSC500-CODE1\"", "collaborators_url"="", "teams_url"=""}, {"ID"="", "node_id"="", "name"="\"P711-LCA-SSC600-CODE1\"", "full_name"="\"P887/P711-LCA-SSC600-CODE1\"", "private"="true", "owner"="", "html_url"="\"https://github.inbcu.com/P887/P711-LCA-SSC600-CODE1\"", "description"="\"Lights Camera Action SAE/SFX SSC\"", "url"="\"https://github.inbcu.com/api/v3/repos/P887/P711-LCA-SSC600-CODE1\"", "collaborators_url"="", "teams_url"=""}, {"ID"="", "node_id"="", "name"="\"P711-LCA-SSC700-CODE1\"", "full_name"="\"P887/P711-LCA-SSC700-CODE1\"", "private"="true", "owner"="", "html_url"="\"https://github.inbcu.com/P887/P711-LCA-SSC700-CODE1\"", "description"="\"Lights Camera Action SAE/SFX SSC\"", "url"="\"https://github.inbcu.com/api/v3/repos/P887/P711-LCA-SSC700-CODE1\"", "collaborators_url"="", "teams_url"=""}, {"ID"="", "node_id"="", "name"="\"P711-LCA-FSC800-CODE1\"", "full_name"="\"P887/P711-LCA-FSC800-CODE1\"", "private"="true", "owner"="", "html_url"="\"https://github.inbcu.com/P887/P711-LCA-FSC800-CODE1\"", "description"="null", "url"="\"https://github.inbcu.com/api/v3/repos/P887/P711-LCA-FSC800-CODE1\"", "collaborators_url"="", "teams_url"=""}, {"ID"="", "node_id"="", "name"="\"P715-LAND-AF-SSC1200-CODE1\"", "full_name"="\"P887/P715-LAND-AF-SSC1200-CODE1\"", "private"="true", "owner"="", "html_url"="\"https://github.inbcu.com/P887/P715-LAND-AF-SSC1200-CODE1\"", "description"="\"Cinnabar\"", "url"="\"https://github.inbcu.com/api/v3/repos/P887/P715-LAND-AF-SSC1200-CODE1\"", "collaborators_url"="", "teams_url"=""}, {"ID"="", "node_id"="", "name"="\"P715-LAND-AF-SSC1400-CODE1\"", "full_name"="\"P887/P715-LAND-AF-SSC1400-CODE1\"", "private"="true", "owner"="", "html_url"="\"https://github.inbcu.com/P887/P715-LAND-AF-SSC1400-CODE1\"", "description"="\"Cinnabar\"", "url"="\"https://github.inbcu.com/api/v3/repos/P887/P715-LAND-AF-SSC1400-CODE1\"", "collaborators_url"="", "teams_url"=""}, {"ID"="", "node_id"="", "name"="\"P715-501A-SSC-0200-CODE1\"", "full_name"="\"P887/P715-501A-SSC-0200-CODE1\"", "private"="true", "owner"="", "html_url"="\"https://github.inbcu.com/P887/P715-501A-SSC-0200-CODE1\"", "description"="\"Cinnabar\"", "url"="\"https://github.inbcu.com/api/v3/repos/P887/P715-501A-SSC-0200-CODE1\"", "collaborators_url"="", "teams_url"=""}, {"ID"="", "node_id"="", "name"="\"P715-501A-SSC-0300-CODE1\"", "full_name"="\"P887/P715-501A-SSC-0300-CODE1\"", "private"="true", "owner"="", "html_url"="\"https://github.inbcu.com/P887/P715-501A-SSC-0300-CODE1\"", "description"="\"Cinnabar\"", "url"="\"https://github.inbcu.com/api/v3/repos/P887/P715-501A-SSC-0300-CODE1\"", "collaborators_url"="", "teams_url"=""}, {"ID"="", "node_id"="", "name"="\"P715-506-SSC-0400-CODE1\"", "full_name"="\"P887/P715-506-SSC-0400-CODE1\"", "private"="true", "owner"="", "html_url"="\"https://github.inbcu.com/P887/P715-506-SSC-0400-CODE1\"", "description"="\"Cinnabar\"", "url"="\"https://github.inbcu.com/api/v3/repos/P887/P715-506-SSC-0400-CODE1\"", "collaborators_url"="", "teams_url"=""}, {"ID"="", "node_id"="", "name"="\"P715-501B-SSC-1200-CODE1\"", "full_name"="\"P887/P715-501B-SSC-1200-CODE1\"", "private"="true", "owner"="", "html_url"="\"https://github.inbcu.com/P887/P715-501B-SSC-1200-CODE1\"", "description"="\"Cinnabar\"", "url"="\"https://github.inbcu.com/api/v3/repos/P887/P715-501B-SSC-1200-CODE1\"", "collaborators_url"="", "teams_url"=""}, {"ID"="", "node_id"="", "name"="\"P715-501A-SSC-1300-CODE1\"", "full_name"="\"P887/P715-501A-SSC-1300-CODE1\"", "private"="true", "owner"="", "html_url"="\"https://github.inbcu.com/P887/P715-501A-SSC-1300-CODE1\"", "description"="\"Cinnabar\"", "url"="\"https://github.inbcu.com/api/v3/repos/P887/P715-501A-SSC-1300-CODE1\"", "collaborators_url"="", "teams_url"=""}, {"ID"="", "node_id"="", "name"="\"P715-501A-SSC-1400-CODE1\"", "full_name"="\"P887/P715-501A-SSC-1400-CODE1\"", "private"="true", "owner"="", "html_url"="\"https://github.inbcu.com/P887/P715-501A-SSC-1400-CODE1\"", "description"="\"Cinnabar\"", "url"="\"https://github.inbcu.com/api/v3/repos/P887/P715-501A-SSC-1400-CODE1\"", "collaborators_url"="", "teams_url"=""}, {"ID"="", "node_id"="", "name"="\"P715-502-SSC-1500-CODE1\"", "full_name"="\"P887/P715-502-SSC-1500-CODE1\"", "private"="true", "owner"="", "html_url"="\"https://github.inbcu.com/P887/P715-502-SSC-1500-CODE1\"", "description"="\"Cinnabar\"", "url"="\"https://github.inbcu.com/api/v3/repos/P887/P715-502-SSC-1500-CODE1\"", "collaborators_url"="", "teams_url"=""}, {"ID"="", "node_id"="", "name"="\"P715-505-SSC-1600-CODE1\"", "full_name"="\"P887/P715-505-SSC-1600-CODE1\"", "private"="true", "owner"="", "html_url"="\"https://github.inbcu.com/P887/P715-505-SSC-1600-CODE1\"", "description"="\"Cinnabar\"", "url"="\"https://github.inbcu.com/api/v3/repos/P887/P715-505-SSC-1600-CODE1\"", "collaborators_url"="", "teams_url"=""}, {"ID"="", "node_id"="", "name"="\"P715-504-SSC-1700-CODE1\"", "full_name"="\"P887/P715-504-SSC-1700-CODE1\"", "private"="true", "owner"="", "html_url"="\"https://github.inbcu.com/P887/P715-504-SSC-1700-CODE1\"", "description"="\"Cinnabar\"", "url"="\"https://github.inbcu.com/api/v3/repos/P887/P715-504-SSC-1700-CODE1\"", "collaborators_url"="", "teams_url"=""}, {"ID"="", "node_id"="", "name"="\"P715-501A-SSC-1800-CODE1\"", "full_name"="\"P887/P715-501A-SSC-1800-CODE1\"", "private"="true", "owner"="", "html_url"="\"https://github.inbcu.com/P887/P715-501A-SSC-1800-CODE1\"", "description"="\"Cinnabar\"", "url"="\"https://github.inbcu.com/api/v3/repos/P887/P715-501A-SSC-1800-CODE1\"", "collaborators_url"="", "teams_url"=""}, {"ID"="", "node_id"="", "name"="\"P715-504-SSC-1900-CODE1\"", "full_name"="\"P887/P715-504-SSC-1900-CODE1\"", "private"="true", "owner"="", "html_url"="\"https://github.inbcu.com/P887/P715-504-SSC-1900-CODE1\"", "description"="\"Cinnabar\"", "url"="\"https://github.inbcu.com/api/v3/repos/P887/P715-504-SSC-1900-CODE1\"", "collaborators_url"="", "teams_url"=""}, {"ID"="", "node_id"="", "name"="\"P715-506-SSC-2400-CODE1\"", "full_name"="\"P887/P715-506-SSC-2400-CODE1\"", "private"="true", "owner"="", "html_url"="\"https://github.inbcu.com/P887/P715-506-SSC-2400-CODE1\"", "description"="\"Cinnabar\"", "url"="\"https://github.inbcu.com/api/v3/repos/P887/P715-506-SSC-2400-CODE1\"", "collaborators_url"="", "teams_url"=""}, {"ID"="", "node_id"="", "name"="\"P715-506-SSC-0500-CODE1\"", "full_name"="\"P887/P715-506-SSC-0500-CODE1\"", "private"="true", "owner"="", "html_url"="\"https://github.inbcu.com/P887/P715-506-SSC-0500-CODE1\"", "description"="\"Animax\"", "url"="\"https://github.inbcu.com/api/v3/repos/P887/P715-506-SSC-0500-CODE1\"", "collaborators_url"="", "teams_url"=""}, {"ID"="", "node_id"="", "name"="\"P715-502-SSC-2000-CODE1\"", "full_name"="\"P887/P715-502-SSC-2000-CODE1\"", "private"="true", "owner"="", "html_url"="\"https://github.inbcu.com/P887/P715-502-SSC-2000-CODE1\"", "description"="\"Animax\"", "url"="\"https://github.inbcu.com/api/v3/repos/P887/P715-502-SSC-2000-CODE1\"", "collaborators_url"="", "teams_url"=""}, {"ID"="", "node_id"="", "name"="\"P715-502-SSC-2100-CODE1\"", "full_name"="\"P887/P715-502-SSC-2100-CODE1\"", "private"="true", "owner"="", "html_url"="\"https://github.inbcu.com/P887/P715-502-SSC-2100-CODE1\"", "description"="\"Animax\"", "url"="\"https://github.inbcu.com/api/v3/repos/P887/P715-502-SSC-2100-CODE1\"", "collaborators_url"="", "teams_url"=""}, {"ID"="", "node_id"="", "name"="\"P715-501B-SSC-2200-CODE1\"", "full_name"="\"P887/P715-501B-SSC-2200-CODE1\"", "private"="true", "owner"="", "html_url"="\"https://github.inbcu.com/P887/P715-501B-SSC-2200-CODE1\"", "description"="\"Animax\"", "url"="\"https://github.inbcu.com/api/v3/repos/P887/P715-501B-SSC-2200-CODE1\"", "collaborators_url"="", "teams_url"=""}, {"ID"="", "node_id"="", "name"="\"P715-501B-SSC-2300-CODE1\"", "full_name"="\"P887/P715-501B-SSC-2300-CODE1\"", "private"="true", "owner"="", "html_url"="\"https://github.inbcu.com/P887/P715-501B-SSC-2300-CODE1\"", "description"="\"Animax\"", "url"="\"https://github.inbcu.com/api/v3/repos/P887/P715-501B-SSC-2300-CODE1\"", "collaborators_url"="", "teams_url"=""}, {"ID"="", "node_id"="", "name"="\"P715-510-SSC-2400-CODE1\"", "full_name"="\"P887/P715-510-SSC-2400-CODE1\"", "private"="true", "owner"="", "html_url"="\"https://github.inbcu.com/P887/P715-510-SSC-2400-CODE1\"", "description"="\"Animax\"", "url"="\"https://github.inbcu.com/api/v3/repos/P887/P715-510-SSC-2400-CODE1\"", "collaborators_url"="", "teams_url"=""}, {"ID"="", "node_id"="", "name"="\"P715-510-SSC-2500-CODE1\"", "full_name"="\"P887/P715-510-SSC-2500-CODE1\"", "private"="true", "owner"="", "html_url"="\"https://github.inbcu.com/P887/P715-510-SSC-2500-CODE1\"", "description"="\"Animax\"", "url"="\"https://github.inbcu.com/api/v3/repos/P887/P715-510-SSC-2500-CODE1\"", "collaborators_url"="", "teams_url"=""}, {"ID"="", "node_id"="", "name"="\"P715-507-SSC-0200-CODE1\"", "full_name"="\"P887/P715-507-SSC-0200-CODE1\"", "private"="true", "owner"="", "html_url"="\"https://github.inbcu.com/P887/P715-507-SSC-0200-CODE1\"", "description"="\"Animax\"", "url"="\"https://github.inbcu.com/api/v3/repos/P887/P715-507-SSC-0200-CODE1\"", "collaborators_url"="", "teams_url"=""}, {"ID"="", "node_id"="", "name"="\"P715-502-SSC-0600-CODE1\"", "full_name"="\"P887/P715-502-SSC-0600-CODE1\"", "private"="true", "owner"="", "html_url"="\"https://github.inbcu.com/P887/P715-502-SSC-0600-CODE1\"", "description"="\"AET\"", "url"="\"https://github.inbcu.com/api/v3/repos/P887/P715-502-SSC-0600-CODE1\"", "collaborators_url"="", "teams_url"=""}, {"ID"="", "node_id"="", "name"="\"P715-501A-SSC-0700-CODE1\"", "full_name"="\"P887/P715-501A-SSC-0700-CODE1\"", "private"="true", "owner"="", "html_url"="\"https://github.inbcu.com/P887/P715-501A-SSC-0700-CODE1\"", "description"="\"AET\"", "url"="\"https://github.inbcu.com/api/v3/repos/P887/P715-501A-SSC-0700-CODE1\"", "collaborators_url"="", "teams_url"=""}, {"ID"="", "node_id"="", "name"="\"P715-501B-SSC-0800-CODE1\"", "full_name"="\"P887/P715-501B-SSC-0800-CODE1\"", "private"="true", "owner"="", "html_url"="\"https://github.inbcu.com/P887/P715-501B-SSC-0800-CODE1\"", "description"="\"AET\"", "url"="\"https://github.inbcu.com/api/v3/repos/P887/P715-501B-SSC-0800-CODE1\"", "collaborators_url"="", "teams_url"=""}, {"ID"="", "node_id"="", "name"="\"P715-505-SSC-0900-CODE1\"", "full_name"="\"P887/P715-505-SSC-0900-CODE1\"", "private"="true", "owner"="", "html_url"="\"https://github.inbcu.com/P887/P715-505-SSC-0900-CODE1\"", "description"="\"AET\"", "url"="\"https://github.inbcu.com/api/v3/repos/P887/P715-505-SSC-0900-CODE1\"", "collaborators_url"="", "teams_url"=""}, {"ID"="", "node_id"="", "name"="\"P715-501A-SSC-1000-CODE1\"", "full_name"="\"P887/P715-501A-SSC-1000-CODE1\"", "private"="true", "owner"="", "html_url"="\"https://github.inbcu.com/P887/P715-501A-SSC-1000-CODE1\"", "description"="\"AET\"", "url"="\"https://github.inbcu.com/api/v3/repos/P887/P715-501A-SSC-1000-CODE1\"", "collaborators_url"="", "teams_url"=""}, {"ID"="", "node_id"="", "name"="\"P715-503-SSC-1100-CODE1\"", "full_name"="\"P887/P715-503-SSC-1100-CODE1\"", "private"="true", "owner"="", "html_url"="\"https://github.inbcu.com/P887/P715-503-SSC-1100-CODE1\"", "description"="\"AET\"", "url"="\"https://github.inbcu.com/api/v3/repos/P887/P715-503-SSC-1100-CODE1\"", "collaborators_url"="", "teams_url"=""}, {"ID"="", "node_id"="", "name"="\"P715-510-SSC-2200-CODE1\"", "full_name"="\"P887/P715-510-SSC-2200-CODE1\"", "private"="true", "owner"="", "html_url"="\"https://github.inbcu.com/P887/P715-510-SSC-2200-CODE1\"", "description"="\"AET\"", "url"="\"https://github.inbcu.com/api/v3/repos/P887/P715-510-SSC-2200-CODE1\"", "collaborators_url"="", "teams_url"=""}, {"ID"="", "node_id"="", "name"="\"P715-510-SSC-2300-CODE1\"", "full_name"="\"P887/P715-510-SSC-2300-CODE1\"", "private"="true", "owner"="", "html_url"="\"https://github.inbcu.com/P887/P715-510-SSC-2300-CODE1\"", "description"="\"AET\"", "url"="\"https://github.inbcu.com/api/v3/repos/P887/P715-510-SSC-2300-CODE1\"", "collaborators_url"="", "teams_url"=""}, {"ID"="", "node_id"="", "name"="\"P712-JWA-CTC-WORKING-DOCS1\"", "full_name"="\"P887/P712-JWA-CTC-WORKING-DOCS1\"", "private"="true", "owner"="", "html_url"="\"https://github.inbcu.com/P887/P712-JWA-CTC-WORKING-DOCS1\"", "description"="\"This repository is to hold all working documents that change frequently throughout comissioning\"", "url"="\"https://github.inbcu.com/api/v3/repos/P887/P712-JWA-CTC-WORKING-DOCS1\"", "collaborators_url"="", "teams_url"=""}, {"ID"="", "node_id"="", "name"="\"P712-JWA-PSM-WORKING-DOCS1\"", "full_name"="\"P887/P712-JWA-PSM-WORKING-DOCS1\"", "private"="true", "owner"="", "html_url"="\"https://github.inbcu.com/P887/P712-JWA-PSM-WORKING-DOCS1\"", "description"="null", "url"="\"https://github.inbcu.com/api/v3/repos/P887/P712-JWA-PSM-WORKING-DOCS1\"", "collaborators_url"="", "teams_url"=""}, {"ID"="", "node_id"="", "name"="\"712-JWA-UC-DOCS1\"", "full_name"="\"P887/712-JWA-UC-DOCS1\"", "private"="true", "owner"="", "html_url"="\"https://github.inbcu.com/P887/712-JWA-UC-DOCS1\"", "description"="\"Intern documents and code for JWA\"", "url"="\"https://github.inbcu.com/api/v3/repos/P887/712-JWA-UC-DOCS1\"", "collaborators_url"="", "teams_url"=""}, {"ID"="", "node_id"="", "name"="\"713-WATERWORLD-SSC100-CODE1\"", "full_name"="\"P887/713-WATERWORLD-SSC100-CODE1\"", "private"="true", "owner"="", "html_url"="\"https://github.inbcu.com/P887/713-WATERWORLD-SSC100-CODE1\"", "description"="\"Birket\"", "url"="\"https://github.inbcu.com/api/v3/repos/P887/713-WATERWORLD-SSC100-CODE1\"", "collaborators_url"="", "teams_url"=""}, {"ID"="", "node_id"="", "name"="\"713-WATERWORLD-SSC200-CODE1\"", "full_name"="\"P887/713-WATERWORLD-SSC200-CODE1\"", "private"="true", "owner"="", "html_url"="\"https://github.inbcu.com/P887/713-WATERWORLD-SSC200-CODE1\"", "description"="\"Tait HPU\"", "url"="\"https://github.inbcu.com/api/v3/repos/P887/713-WATERWORLD-SSC200-CODE1\"", "collaborators_url"="", "teams_url"=""}, {"ID"="", "node_id"="", "name"="\"713-WATERWORLD-SSC300-CODE1\"", "full_name"="\"P887/713-WATERWORLD-SSC300-CODE1\"", "private"="true", "owner"="", "html_url"="\"https://github.inbcu.com/P887/713-WATERWORLD-SSC300-CODE1\"", "description"="\"HXT ATOL Gates\"", "url"="\"https://github.inbcu.com/api/v3/repos/P887/713-WATERWORLD-SSC300-CODE1\"", "collaborators_url"="", "teams_url"=""}, {"ID"="", "node_id"="", "name"="\"P713-WATERWORLD-SSC400-CODE1\"", "full_name"="\"P887/P713-WATERWORLD-SSC400-CODE1\"", "private"="true", "owner"="", "html_url"="\"https://github.inbcu.com/P887/P713-WATERWORLD-SSC400-CODE1\"", "description"="\"Tasc Flame\"", "url"="\"https://github.inbcu.com/api/v3/repos/P887/P713-WATERWORLD-SSC400-CODE1\"", "collaborators_url"="", "teams_url"=""}, {"ID"="", "node_id"="", "name"="\"P713-WATERWORLD-SSC500-CODE1\"", "full_name"="\"P887/P713-WATERWORLD-SSC500-CODE1\"", "private"="true", "owner"="", "html_url"="\"https://github.inbcu.com/P887/P713-WATERWORLD-SSC500-CODE1\"", "description"="\"TAIT Collapsing Tower\"", "url"="\"https://github.inbcu.com/api/v3/repos/P887/P713-WATERWORLD-SSC500-CODE1\"", "collaborators_url"="", "teams_url"=""}, {"ID"="", "node_id"="", "name"="\"P713-WATERWORLD-SSC600-CODE1\"", "full_name"="\"P887/P713-WATERWORLD-SSC600-CODE1\"", "private"="true", "owner"="", "html_url"="\"https://github.inbcu.com/P887/P713-WATERWORLD-SSC600-CODE1\"", "description"="\"TAIT Mariner Counterweight\"", "url"="\"https://github.inbcu.com/api/v3/repos/P887/P713-WATERWORLD-SSC600-CODE1\"", "collaborators_url"="", "teams_url"=""}, {"ID"="", "node_id"="", "name"="\"P713-WATERWORLD-SSC700-CODE1\"", "full_name"="\"P887/P713-WATERWORLD-SSC700-CODE1\"", "private"="true", "owner"="", "html_url"="\"https://github.inbcu.com/P887/P713-WATERWORLD-SSC700-CODE1\"", "description"="\"AET Type 1 and 2 Effects\"", "url"="\"https://github.inbcu.com/api/v3/repos/P887/P713-WATERWORLD-SSC700-CODE1\"", "collaborators_url"="", "teams_url"=""}, {"ID"="", "node_id"="", "name"="\"P713-WATERWORLD-SSC710-CODE1\"", "full_name"="\"P887/P713-WATERWORLD-SSC710-CODE1\"", "private"="true", "owner"="", "html_url"="\"https://github.inbcu.com/P887/P713-WATERWORLD-SSC710-CODE1\"", "description"="\"AET Type 1 and 2 effects\"", "url"="\"https://github.inbcu.com/api/v3/repos/P887/P713-WATERWORLD-SSC710-CODE1\"", "collaborators_url"="", "teams_url"=""}, {"ID"="", "node_id"="", "name"="\"P713-WATERWORLD-SSC4000-CODE1\"", "full_name"="\"P887/P713-WATERWORLD-SSC4000-CODE1\"", "private"="true", "owner"="", "html_url"="\"https://github.inbcu.com/P887/P713-WATERWORLD-SSC4000-CODE1\"", "description"="\"Technomedia AV\"", "url"="\"https://github.inbcu.com/api/v3/repos/P887/P713-WATERWORLD-SSC4000-CODE1\"", "collaborators_url"="", "teams_url"=""}, {"ID"="", "node_id"="", "name"="\"P713-WATERWORLD-SSC800-CODE1\"", "full_name"="\"P887/P713-WATERWORLD-SSC800-CODE1\"", "private"="true", "owner"="", "html_url"="\"https://github.inbcu.com/P887/P713-WATERWORLD-SSC800-CODE1\"", "description"="\"Birket Pyro Control\"", "url"="\"https://github.inbcu.com/api/v3/repos/P887/P713-WATERWORLD-SSC800-CODE1\"", "collaborators_url"="", "teams_url"=""}, {"ID"="", "node_id"="", "name"="\"P717-MM-LCT-CODE1\"", "full_name"="\"P887/P717-MM-LCT-CODE1\"", "private"="true", "owner"="", "html_url"="\"https://github.inbcu.com/P887/P717-MM-LCT-CODE1\"", "description"="\"Live Character Theater (BIRKET)\"", "url"="\"https://github.inbcu.com/api/v3/repos/P887/P717-MM-LCT-CODE1\"", "collaborators_url"="", "teams_url"=""}, {"ID"="", "node_id"="", "name"="\"P712-JWA-RCS-200-300-ADD-REMOVE-TS-CODE1\"", "full_name"="\"P887/P712-JWA-RCS-200-300-ADD-REMOVE-TS-CODE1\"", "private"="true", "owner"="", "html_url"="\"https://github.inbcu.com/P887/P712-JWA-RCS-200-300-ADD-REMOVE-TS-CODE1\"", "description"="null", "url"="\"https://github.inbcu.com/api/v3/repos/P887/P712-JWA-RCS-200-300-ADD-REMOVE-TS-CODE1\"", "collaborators_url"="", "teams_url"=""}, {"ID"="", "node_id"="", "name"="\"P712-RCS-400-500-IB-TS-CODE1\"", "full_name"="\"P887/P712-RCS-400-500-IB-TS-CODE1\"", "private"="true", "owner"="", "html_url"="\"https://github.inbcu.com/P887/P712-RCS-400-500-IB-TS-CODE1\"", "description"="null", "url"="\"https://github.inbcu.com/api/v3/repos/P887/P712-RCS-400-500-IB-TS-CODE1\"", "collaborators_url"="", "teams_url"=""}, {"ID"="", "node_id"="", "name"="\"P712_TEST_REPO\"", "full_name"="\"P887/P712_TEST_REPO\"", "private"="true", "owner"="", "html_url"="\"https://github.inbcu.com/P887/P712_TEST_REPO\"", "description"="\"Used to test front end communication with corporate GIT\"", "url"="\"https://github.inbcu.com/api/v3/repos/P887/P712_TEST_REPO\"", "collaborators_url"="", "teams_url"=""}, {"ID"="", "node_id"="", "name"="\"P712-JWA-CABIN-CODE1\"", "full_name"="\"P887/P712-JWA-CABIN-CODE1\"", "private"="true", "owner"="", "html_url"="\"https://github.inbcu.com/P887/P712-JWA-CABIN-CODE1\"", "description"="null", "url"="\"https://github.inbcu.com/api/v3/repos/P887/P712-JWA-CABIN-CODE1\"", "collaborators_url"="", "teams_url"=""}, {"ID"="", "node_id"="", "name"="\"P712-Test-HG-Tracking\"", "full_name"="\"P887/P712-Test-HG-Tracking\"", "private"="true", "owner"="", "html_url"="\"https://github.inbcu.com/P887/P712-Test-HG-Tracking\"", "description"="null", "url"="\"https://github.inbcu.com/api/v3/repos/P887/P712-Test-HG-Tracking\"", "collaborators_url"="", "teams_url"=""}, {"ID"="", "node_id"="", "name"="\"P717-703-LCT-CODE1\"", "full_name"="\"P887/P717-703-LCT-CODE1\"", "private"="true", "owner"="", "html_url"="\"https://github.inbcu.com/P887/P717-703-LCT-CODE1\"", "description"="\"Live Character Theater\"", "url"="\"https://github.inbcu.com/api/v3/repos/P887/P717-703-LCT-CODE1\"", "collaborators_url"="", "teams_url"=""}, {"ID"="", "node_id"="", "name"="\"P716-P557-TRANSFORMERS-RV-MASTER-CODE1\"", "full_name"="\"P887/P716-P557-TRANSFORMERS-RV-MASTER-CODE1\"", "private"="true", "owner"="", "html_url"="\"https://github.inbcu.com/P887/P716-P557-TRANSFORMERS-RV-MASTER-CODE1\"", "description"="null", "url"="\"https://github.inbcu.com/api/v3/repos/P887/P716-P557-TRANSFORMERS-RV-MASTER-CODE1\"", "collaborators_url"="", "teams_url"=""}, {"ID"="", "node_id"="", "name"="\"P715-FJ-WORKING-DOCS1\"", "full_name"="\"P887/P715-FJ-WORKING-DOCS1\"", "private"="true", "owner"="", "html_url"="\"https://github.inbcu.com/P887/P715-FJ-WORKING-DOCS1\"", "description"="\"Working docs for FJ \"", "url"="\"https://github.inbcu.com/api/v3/repos/P887/P715-FJ-WORKING-DOCS1\"", "collaborators_url"="", "teams_url"=""}, {"ID"="", "node_id"="", "name"="\"P719-SSIP-CODE1\"", "full_name"="\"P887/P719-SSIP-CODE1\"", "private"="true", "owner"="", "html_url"="\"https://github.inbcu.com/P887/P719-SSIP-CODE1\"", "description"="null", "url"="\"https://github.inbcu.com/api/v3/repos/P887/P719-SSIP-CODE1\"", "collaborators_url"="", "teams_url"=""}, {"ID"="", "node_id"="", "name"="\"P712-JWA-FAT-Track-Code1\"", "full_name"="\"P887/P712-JWA-FAT-Track-Code1\"", "private"="true", "owner"="", "html_url"="\"https://github.inbcu.com/P887/P712-JWA-FAT-Track-Code1\"", "description"="null", "url"="\"https://github.inbcu.com/api/v3/repos/P887/P712-JWA-FAT-Track-Code1\"", "collaborators_url"="", "teams_url"=""}, {"ID"="", "node_id"="", "name"="\"712-JWA-RCS-SIM-CODE1\"", "full_name"="\"P887/712-JWA-RCS-SIM-CODE1\"", "private"="true", "owner"="", "html_url"="\"https://github.inbcu.com/P887/712-JWA-RCS-SIM-CODE1\"", "description"="null", "url"="\"https://github.inbcu.com/api/v3/repos/P887/712-JWA-RCS-SIM-CODE1\"", "collaborators_url"="", "teams_url"=""}, {"ID"="", "node_id"="", "name"="\"P716-TRANSFORMERS-EVAC-CODE1\"", "full_name"="\"P887/P716-TRANSFORMERS-EVAC-CODE1\"", "private"="true", "owner"="", "html_url"="\"https://github.inbcu.com/P887/P716-TRANSFORMERS-EVAC-CODE1\"", "description"="null", "url"="\"https://github.inbcu.com/api/v3/repos/P887/P716-TRANSFORMERS-EVAC-CODE1\"", "collaborators_url"="", "teams_url"=""}, {"ID"="", "node_id"="", "name"="\"P716-TRANSFORMERS-SSC2100-CODE1\"", "full_name"="\"P887/P716-TRANSFORMERS-SSC2100-CODE1\"", "private"="true", "owner"="", "html_url"="\"https://github.inbcu.com/P887/P716-TRANSFORMERS-SSC2100-CODE1\"", "description"="null", "url"="\"https://github.inbcu.com/api/v3/repos/P887/P716-TRANSFORMERS-SSC2100-CODE1\"", "collaborators_url"="", "teams_url"=""}, {"ID"="", "node_id"="", "name"="\"P712-JWA-RCS-Sim-Release\"", "full_name"="\"P887/P712-JWA-RCS-Sim-Release\"", "private"="true", "owner"="", "html_url"="\"https://github.inbcu.com/P887/P712-JWA-RCS-Sim-Release\"", "description"="null", "url"="\"https://github.inbcu.com/api/v3/repos/P887/P712-JWA-RCS-Sim-Release\"", "collaborators_url"="", "teams_url"=""}, {"ID"="", "node_id"="", "name"="\"P711-MPT-SCS2000-CODE1\"", "full_name"="\"P887/P711-MPT-SCS2000-CODE1\"", "private"="true", "owner"="", "html_url"="\"https://github.inbcu.com/P887/P711-MPT-SCS2000-CODE1\"", "description"="\"Show System Controller – Show head end (Navigator) (Tait)\"", "url"="\"https://github.inbcu.com/api/v3/repos/P887/P711-MPT-SCS2000-CODE1\"", "collaborators_url"="", "teams_url"=""}, {"ID"="", "node_id"="", "name"="\"P711-MPT-SSC200-CODE1\"", "full_name"="\"P887/P711-MPT-SSC200-CODE1\"", "private"="true", "owner"="", "html_url"="\"https://github.inbcu.com/P887/P711-MPT-SSC200-CODE1\"", "description"="\"FoH/BoH Overhead Rigging Systems (Tait)  *FoH = Front of House, BoH = Back of House\"", "url"="\"https://github.inbcu.com/api/v3/repos/P887/P711-MPT-SSC200-CODE1\"", "collaborators_url"="", "teams_url"=""}, {"ID"="", "node_id"="", "name"="\"P711-MPT-SSC300-CODE1\"", "full_name"="\"P887/P711-MPT-SSC300-CODE1\"", "private"="true", "owner"="", "html_url"="\"https://github.inbcu.com/P887/P711-MPT-SSC300-CODE1\"", "description"="\"Stage/Scenic Automation Controller (Tait)\"", "url"="\"https://github.inbcu.com/api/v3/repos/P887/P711-MPT-SSC300-CODE1\"", "collaborators_url"="", "teams_url"=""}, {"ID"="", "node_id"="", "name"="\"P711-MPT-SSC400-CODE1\"", "full_name"="\"P887/P711-MPT-SSC400-CODE1\"", "private"="true", "owner"="", "html_url"="\"https://github.inbcu.com/P887/P711-MPT-SSC400-CODE1\"", "description"="\"Stage Lift System (JV contracted vendor – not yet identified)\"", "url"="\"https://github.inbcu.com/api/v3/repos/P887/P711-MPT-SSC400-CODE1\"", "collaborators_url"="", "teams_url"=""}, {"ID"="", "node_id"="", "name"="\"P711-MPT-SSC600-CODE1\"", "full_name"="\"P887/P711-MPT-SSC600-CODE1\"", "private"="true", "owner"="", "html_url"="\"https://github.inbcu.com/P887/P711-MPT-SSC600-CODE1\"", "description"="\"Flying Dragon Animated Figure (CTC)\"", "url"="\"https://github.inbcu.com/api/v3/repos/P887/P711-MPT-SSC600-CODE1\"", "collaborators_url"="", "teams_url"=""}, {"ID"="", "node_id"="", "name"="\"P711-MPT-SSC700-CODE1\"", "full_name"="\"P887/P711-MPT-SSC700-CODE1\"", "private"="true", "owner"="", "html_url"="\"https://github.inbcu.com/P887/P711-MPT-SSC700-CODE1\"", "description"="\"Stage Dragon Animated Figure (CTC)\"", "url"="\"https://github.inbcu.com/api/v3/repos/P887/P711-MPT-SSC700-CODE1\"", "collaborators_url"="", "teams_url"=""}, {"ID"="", "node_id"="", "name"="\"P711-MPT-SSC1000-CODE1\"", "full_name"="\"P887/P711-MPT-SSC1000-CODE1\"", "private"="true", "owner"="", "html_url"="\"https://github.inbcu.com/P887/P711-MPT-SSC1000-CODE1\"", "description"="\"Creature Master Sub-System Controller (CTC)\"", "url"="\"https://github.inbcu.com/api/v3/repos/P887/P711-MPT-SSC1000-CODE1\"", "collaborators_url"="", "teams_url"=""}, {"ID"="", "node_id"="", "name"="\"P717-MM-RCS-CODE2\"", "full_name"="\"P887/P717-MM-RCS-CODE2\"", "private"="true", "owner"="", "html_url"="\"https://github.inbcu.com/P887/P717-MM-RCS-CODE2\"", "description"="\"Minion Mayhem Repository number 2, continuation of P717-MM-RCS-CODE1 after size limit\"", "url"="\"https://github.inbcu.com/api/v3/repos/P887/P717-MM-RCS-CODE2\"", "collaborators_url"="", "teams_url"=""}, {"ID"="", "node_id"="", "name"="\"P711-MPT-SSC1100-CODE1\"", "full_name"="\"P887/P711-MPT-SSC1100-CODE1\"", "private"="true", "owner"="", "html_url"="\"https://github.inbcu.com/P887/P711-MPT-SSC1100-CODE1\"", "description"="\"BSD Fire Curtain SSC\"", "url"="\"https://github.inbcu.com/api/v3/repos/P887/P711-MPT-SSC1100-CODE1\"", "collaborators_url"="", "teams_url"=""}, {"ID"="", "node_id"="", "name"="\"P711-MPT-SSC1200-CODE1\"", "full_name"="\"P887/P711-MPT-SSC1200-CODE1\"", "private"="true", "owner"="", "html_url"="\"https://github.inbcu.com/P887/P711-MPT-SSC1200-CODE1\"", "description"="\"BSD Speaker Hoist Rigging System\"", "url"="\"https://github.inbcu.com/api/v3/repos/P887/P711-MPT-SSC1200-CODE1\"", "collaborators_url"="", "teams_url"=""}, {"ID"="", "node_id"="", "name"="\"P716-DECEPTICOASTER-DRIVEA-CODE1\"", "full_name"="\"P887/P716-DECEPTICOASTER-DRIVEA-CODE1\"", "private"="true", "owner"="", "html_url"="\"https://github.inbcu.com/P887/P716-DECEPTICOASTER-DRIVEA-CODE1\"", "description"="\"Drives A SSC - Altec\"", "url"="\"https://github.inbcu.com/api/v3/repos/P887/P716-DECEPTICOASTER-DRIVEA-CODE1\"", "collaborators_url"="", "teams_url"=""}, {"ID"="", "node_id"="", "name"="\"P716-DECEPTICOASTER-DRIVEB-CODE1\"", "full_name"="\"P887/P716-DECEPTICOASTER-DRIVEB-CODE1\"", "private"="true", "owner"="", "html_url"="\"https://github.inbcu.com/P887/P716-DECEPTICOASTER-DRIVEB-CODE1\"", "description"="\"Drives B SSC - Altec\"", "url"="\"https://github.inbcu.com/api/v3/repos/P887/P716-DECEPTICOASTER-DRIVEB-CODE1\"", "collaborators_url"="", "teams_url"=""}, {"ID"="", "node_id"="", "name"="\"P716-DECEPTICOASTER-MGS-CODE1\"", "full_name"="\"P887/P716-DECEPTICOASTER-MGS-CODE1\"", "private"="true", "owner"="", "html_url"="\"https://github.inbcu.com/P887/P716-DECEPTICOASTER-MGS-CODE1\"", "description"="\"MGs - Altec\"", "url"="\"https://github.inbcu.com/api/v3/repos/P887/P716-DECEPTICOASTER-MGS-CODE1\"", "collaborators_url"="", "teams_url"=""}, {"ID"="", "node_id"="", "name"="\"P712-JFLYER-VCS-CODE1\"", "full_name"="\"P887/P712-JFLYER-VCS-CODE1\"", "private"="true", "owner"="", "html_url"="\"https://github.inbcu.com/P887/P712-JFLYER-VCS-CODE1\"", "description"="\"MACK J-Flyer Vehicle Code Repository\"", "url"="\"https://github.inbcu.com/api/v3/repos/P887/P712-JFLYER-VCS-CODE1\"", "collaborators_url"="", "teams_url"=""}, {"ID"="", "node_id"="", "name"="\"P715-FJ-HMI-CODE1\"", "full_name"="\"P887/P715-FJ-HMI-CODE1\"", "private"="true", "owner"="", "html_url"="\"https://github.inbcu.com/P887/P715-FJ-HMI-CODE1\"", "description"="\"FJ HMI\"", "url"="\"https://github.inbcu.com/api/v3/repos/P887/P715-FJ-HMI-CODE1\"", "collaborators_url"="", "teams_url"=""}, {"ID"="", "node_id"="", "name"="\"P714-SSC-2100-SFX-FOG-CODE1\"", "full_name"="\"P887/P714-SSC-2100-SFX-FOG-CODE1\"", "private"="true", "owner"="", "html_url"="\"https://github.inbcu.com/P887/P714-SSC-2100-SFX-FOG-CODE1\"", "description"="\"KFP Type 2 SFX/FOG SSC 2100\"", "url"="\"https://github.inbcu.com/api/v3/repos/P887/P714-SSC-2100-SFX-FOG-CODE1\"", "collaborators_url"="", "teams_url"=""}, {"ID"="", "node_id"="", "name"="\"P714-SSC-2200-SFX-FOG-CODE1\"", "full_name"="\"P887/P714-SSC-2200-SFX-FOG-CODE1\"", "private"="true", "owner"="", "html_url"="\"https://github.inbcu.com/P887/P714-SSC-2200-SFX-FOG-CODE1\"", "description"="\"KFP Type 2 SSC 2200 SFX/FOG\"", "url"="\"https://github.inbcu.com/api/v3/repos/P887/P714-SSC-2200-SFX-FOG-CODE1\"", "collaborators_url"="", "teams_url"=""}, {"ID"="", "node_id"="", "name"="\"P711-114-GRONCKLES-CODE1\"", "full_name"="\"P887/P711-114-GRONCKLES-CODE1\"", "private"="true", "owner"="", "html_url"="\"https://github.inbcu.com/P887/P711-114-GRONCKLES-CODE1\"", "description"="\"Animated Figures\"", "url"="\"https://github.inbcu.com/api/v3/repos/P887/P711-114-GRONCKLES-CODE1\"", "collaborators_url"="", "teams_url"=""}, {"ID"="", "node_id"="", "name"="\"P719-PONY-SSC-602-101-1-CODE1\"", "full_name"="\"P887/P719-PONY-SSC-602-101-1-CODE1\"", "private"="true", "owner"="", "html_url"="\"https://github.inbcu.com/P887/P719-PONY-SSC-602-101-1-CODE1\"", "description"="\"Pony Float 1\"", "url"="\"https://github.inbcu.com/api/v3/repos/P887/P719-PONY-SSC-602-101-1-CODE1\"", "collaborators_url"="", "teams_url"=""}, {"ID"="", "node_id"="", "name"="\"P719-PONY-SSC-602-101-2-CODE1\"", "full_name"="\"P887/P719-PONY-SSC-602-101-2-CODE1\"", "private"="true", "owner"="", "html_url"="\"https://github.inbcu.com/P887/P719-PONY-SSC-602-101-2-CODE1\"", "description"="\"Pony Float 2\"", "url"="\"https://github.inbcu.com/api/v3/repos/P887/P719-PONY-SSC-602-101-2-CODE1\"", "collaborators_url"="", "teams_url"=""}, {"ID"="", "node_id"="", "name"="\"P719-PONY-SSC-602-101-3-CODE1\"", "full_name"="\"P887/P719-PONY-SSC-602-101-3-CODE1\"", "private"="true", "owner"="", "html_url"="\"https://github.inbcu.com/P887/P719-PONY-SSC-602-101-3-CODE1\"", "description"="\"Pony Float 3\"", "url"="\"https://github.inbcu.com/api/v3/repos/P887/P719-PONY-SSC-602-101-3-CODE1\"", "collaborators_url"="", "teams_url"=""}, {"ID"="", "node_id"="", "name"="\"P719-LANTERN-SSC-602-104-CODE1\"", "full_name"="\"P887/P719-LANTERN-SSC-602-104-CODE1\"", "private"="true", "owner"="", "html_url"="\"https://github.inbcu.com/P887/P719-LANTERN-SSC-602-104-CODE1\"", "description"="\"Lantern Float\"", "url"="\"https://github.inbcu.com/api/v3/repos/P887/P719-LANTERN-SSC-602-104-CODE1\"", "collaborators_url"="", "teams_url"=""}, {"ID"="", "node_id"="", "name"="\"P719-LANTERN-SSC-602-105-CODE1\"", "full_name"="\"P887/P719-LANTERN-SSC-602-105-CODE1\"", "private"="true", "owner"="", "html_url"="\"https://github.inbcu.com/P887/P719-LANTERN-SSC-602-105-CODE1\"", "description"="\"Lantern Float Secondary Drive\"", "url"="\"https://github.inbcu.com/api/v3/repos/P887/P719-LANTERN-SSC-602-105-CODE1\"", "collaborators_url"="", "teams_url"=""}, {"ID"="", "node_id"="", "name"="\"P719-SUPER-SILLY-SSC-602-103-CODE1\"", "full_name"="\"P887/P719-SUPER-SILLY-SSC-602-103-CODE1\"", "private"="true", "owner"="", "html_url"="\"https://github.inbcu.com/P887/P719-SUPER-SILLY-SSC-602-103-CODE1\"", "description"="\"Super Silly Float\"", "url"="\"https://github.inbcu.com/api/v3/repos/P887/P719-SUPER-SILLY-SSC-602-103-CODE1\"", "collaborators_url"="", "teams_url"=""}, {"ID"="", "node_id"="", "name"="\"P719-SPACEKILLERS-SSC-602-103-CODE1\"", "full_name"="\"P887/P719-SPACEKILLERS-SSC-602-103-CODE1\"", "private"="true", "owner"="", "html_url"="\"https://github.inbcu.com/P887/P719-SPACEKILLERS-SSC-602-103-CODE1\"", "description"="null", "url"="\"https://github.inbcu.com/api/v3/repos/P887/P719-SPACEKILLERS-SSC-602-103-CODE1\"", "collaborators_url"="", "teams_url"=""}, {"ID"="", "node_id"="", "name"="\"P719-YELLOWCART-SSC-602-104-CODE1\"", "full_name"="\"P887/P719-YELLOWCART-SSC-602-104-CODE1\"", "private"="true", "owner"="", "html_url"="\"https://github.inbcu.com/P887/P719-YELLOWCART-SSC-602-104-CODE1\"", "description"="\"Yellow Cart\"", "url"="\"https://github.inbcu.com/api/v3/repos/P887/P719-YELLOWCART-SSC-602-104-CODE1\"", "collaborators_url"="", "teams_url"=""}, {"ID"="", "node_id"="", "name"="\"P719-ONIONCOACH-SSC-602-103-CODE1\"", "full_name"="\"P887/P719-ONIONCOACH-SSC-602-103-CODE1\"", "private"="true", "owner"="", "html_url"="\"https://github.inbcu.com/P887/P719-ONIONCOACH-SSC-602-103-CODE1\"", "description"="\"Onion Coach\"", "url"="\"https://github.inbcu.com/api/v3/repos/P887/P719-ONIONCOACH-SSC-602-103-CODE1\"", "collaborators_url"="", "teams_url"=""}, {"ID"="", "node_id"="", "name"="\"P719-SHREK-SSC-602-103-CODE1\"", "full_name"="\"P887/P719-SHREK-SSC-602-103-CODE1\"", "private"="true", "owner"="", "html_url"="\"https://github.inbcu.com/P887/P719-SHREK-SSC-602-103-CODE1\"", "description"="\"Shrek's Castle\"", "url"="\"https://github.inbcu.com/api/v3/repos/P887/P719-SHREK-SSC-602-103-CODE1\"", "collaborators_url"="", "teams_url"=""}, {"ID"="", "node_id"="", "name"="\"P719-UNICYCLE1-SSC-602-106-CODE1\"", "full_name"="\"P887/P719-UNICYCLE1-SSC-602-106-CODE1\"", "private"="true", "owner"="", "html_url"="\"https://github.inbcu.com/P887/P719-UNICYCLE1-SSC-602-106-CODE1\"", "description"="\"Unicycle 1\"", "url"="\"https://github.inbcu.com/api/v3/repos/P887/P719-UNICYCLE1-SSC-602-106-CODE1\"", "collaborators_url"="", "teams_url"=""}, {"ID"="", "node_id"="", "name"="\"P719-UNICYCLE2-SSC-602-106-CODE1\"", "full_name"="\"P887/P719-UNICYCLE2-SSC-602-106-CODE1\"", "private"="true", "owner"="", "html_url"="\"https://github.inbcu.com/P887/P719-UNICYCLE2-SSC-602-106-CODE1\"", "description"="\"Unicycle 2\"", "url"="\"https://github.inbcu.com/api/v3/repos/P887/P719-UNICYCLE2-SSC-602-106-CODE1\"", "collaborators_url"="", "teams_url"=""}, {"ID"="", "node_id"="", "name"="\"P719-UNICYCLE3-SSC-602-106-CODE1\"", "full_name"="\"P887/P719-UNICYCLE3-SSC-602-106-CODE1\"", "private"="true", "owner"="", "html_url"="\"https://github.inbcu.com/P887/P719-UNICYCLE3-SSC-602-106-CODE1\"", "description"="\"Unicycle 3\"", "url"="\"https://github.inbcu.com/api/v3/repos/P887/P719-UNICYCLE3-SSC-602-106-CODE1\"", "collaborators_url"="", "teams_url"=""}, {"ID"="", "node_id"="", "name"="\"P719-UNICYCLE4-SSC-602-106-CODE1\"", "full_name"="\"P887/P719-UNICYCLE4-SSC-602-106-CODE1\"", "private"="true", "owner"="", "html_url"="\"https://github.inbcu.com/P887/P719-UNICYCLE4-SSC-602-106-CODE1\"", "description"="\"Unicycle 4\"", "url"="\"https://github.inbcu.com/api/v3/repos/P887/P719-UNICYCLE4-SSC-602-106-CODE1\"", "collaborators_url"="", "teams_url"=""}, {"ID"="", "node_id"="", "name"="\"P719-GLORIAS-SSC-602-103-CODE1\"", "full_name"="\"P887/P719-GLORIAS-SSC-602-103-CODE1\"", "private"="true", "owner"="", "html_url"="\"https://github.inbcu.com/P887/P719-GLORIAS-SSC-602-103-CODE1\"", "description"="\"Gloria's Balloon\"", "url"="\"https://github.inbcu.com/api/v3/repos/P887/P719-GLORIAS-SSC-602-103-CODE1\"", "collaborators_url"="", "teams_url"=""}, {"ID"="", "node_id"="", "name"="\"P719-JULIEN-SSC-602-102-CODE1\"", "full_name"="\"P887/P719-JULIEN-SSC-602-102-CODE1\"", "private"="true", "owner"="", "html_url"="\"https://github.inbcu.com/P887/P719-JULIEN-SSC-602-102-CODE1\"", "description"="\"King Julien\"", "url"="\"https://github.inbcu.com/api/v3/repos/P887/P719-JULIEN-SSC-602-102-CODE1\"", "collaborators_url"="", "teams_url"=""}, {"ID"="", "node_id"="", "name"="\"P719-AFROCIRCUS-SSC-602-103-CODE1\"", "full_name"="\"P887/P719-AFROCIRCUS-SSC-602-103-CODE1\"", "private"="true", "owner"="", "html_url"="\"https://github.inbcu.com/P887/P719-AFROCIRCUS-SSC-602-103-CODE1\"", "description"="\"Afro Circus Tent\"", "url"="\"https://github.inbcu.com/api/v3/repos/P887/P719-AFROCIRCUS-SSC-602-103-CODE1\"", "collaborators_url"="", "teams_url"=""}, {"ID"="", "node_id"="", "name"="\"P719-MRPING-SSC-602-102-CODE1\"", "full_name"="\"P887/P719-MRPING-SSC-602-102-CODE1\"", "private"="true", "owner"="", "html_url"="\"https://github.inbcu.com/P887/P719-MRPING-SSC-602-102-CODE1\"", "description"="\"Mr. Ping\"", "url"="\"https://github.inbcu.com/api/v3/repos/P887/P719-MRPING-SSC-602-102-CODE1\"", "collaborators_url"="", "teams_url"=""}, {"ID"="", "node_id"="", "name"="\"P719-MASTEROX-SSC-602-103-CODE1\"", "full_name"="\"P887/P719-MASTEROX-SSC-602-103-CODE1\"", "private"="true", "owner"="", "html_url"="\"https://github.inbcu.com/P887/P719-MASTEROX-SSC-602-103-CODE1\"", "description"="\"Master Ox\"", "url"="\"https://github.inbcu.com/api/v3/repos/P887/P719-MASTEROX-SSC-602-103-CODE1\"", "collaborators_url"="", "teams_url"=""}, {"ID"="", "node_id"="", "name"="\"P719-JADE-SSC-602-104-CODE1\"", "full_name"="\"P887/P719-JADE-SSC-602-104-CODE1\"", "private"="true", "owner"="", "html_url"="\"https://github.inbcu.com/P887/P719-JADE-SSC-602-104-CODE1\"", "description"="\"Jade Palace\"", "url"="\"https://github.inbcu.com/api/v3/repos/P887/P719-JADE-SSC-602-104-CODE1\"", "collaborators_url"="", "teams_url"=""}, {"ID"="", "node_id"="", "name"="\"P719-JADE-SSC-602--106-CODE1\"", "full_name"="\"P887/P719-JADE-SSC-602--106-CODE1\"", "private"="true", "owner"="", "html_url"="\"https://github.inbcu.com/P887/P719-JADE-SSC-602--106-CODE1\"", "description"="\"Jade Palace Drive\"", "url"="\"https://github.inbcu.com/api/v3/repos/P887/P719-JADE-SSC-602--106-CODE1\"", "collaborators_url"="", "teams_url"=""}] ("Repos")
  n1 = call "Git-Enterprise-Register Git Client with Authentication.vi"("Postman Hash"="MjA2NDE3NTU5OjJmYTJkNzNmODIzOTI5MTQ0YmM3NjEzOWE1NmE1NmZhMmRhNzVkNGI=" ("value")) -> ("error out"=w1:errorcluster, "Refnum out"=w5:T2)  [unwired: 9 in]
  n2 = call "Git-Enterprise-Get All Repos In Org.vi"("Error In"=w1, "Organization"="Organization", "Server"="Server", "Refnum in"=w5) -> ("Repos"=w6:T1[])  [unwired: 6 in, 1 out]
  n3 = flat-sequence {
    tunnel: w6 -> [_]
    frame #0 {
    }
  }
